vi "XW angle calib checker_Psi_k_PN.vi"(0 "XW_Calib_Map file path (dialog if empty)":path=path "C:/Documents and Settings/Paul Nathan/Desktop/XW Calib Map/XW angle calib checker/XW002_OH74.txt") -> (1 "Quantities that vary with Uref (epsilon, theta, k) (higher order method)":string="Uref (m/s)\teps1 (deg)\teps2 (deg)\tProbe zero err. (deg)\ttheta 1 (deg)\ttheta 2 (deg)\tk1\tk2\r\n0.5018157894736842\t6.6267533355295098\t-2.9096917617315157\t1.8585307868989971\t-71.8440498634698059\t62.9636877172930269\t0.6599332295131556\t0.5182677319056693\r\n0.9994315789473684\t-1.5238812538483015\t0.9867720938009503\t-0.2685545800236756\t-50.7967211983630804\t49.0160971121406277\t0.4477378321660210\t0.4147363151308795\r\n2.0002052631578948\t-0.7133248964583321\t0.8757082064818565\t0.0811916550117622\t-47.4142025982968249\t46.7238739777964795\t0.3482854524979783\t0.3208003585595113\r\n3.0007842105263158\t0.1760631838109192\t0.0773496663189750\t0.1267064250649471\t-46.5210606369966655\t46.4000168794064791\t0.3180701353043149\t0.2880980466431171\r\n3.9999473684210529\t0.1906487887884856\t-0.2531251578949707\t-0.0312381845532425\t-46.1290205114913973\t46.2520699692747428\t0.2973863116337985\t0.2724916341605894\r\n4.9998315789473686\t0.2282387696125578\t-0.2130683224321221\t0.0075852235902178\t-45.8252448288331848\t46.0312176850919527\t0.2848963782809627\t0.2591128097080996\r\n6.9997315789473680\t0.1263159354503486\t-0.1724714828642656\t-0.0230777737069585\t-45.2896437061695636\t45.4966612147379905\t0.2642800771604700\t0.2410224971037092\r\n9.0019315789473691\t-0.0565462004426682\t0.0773785766074348\t0.0104161880823833\t-44.8675096760090781\t45.0959281609883007\t0.2463064031896132\t0.2236365187658773\r\n10.9999736842105253\t-0.2539290822848189\t0.4859354251419680\t0.1160031714285746\t-44.4053231675819475\t44.4986166412718447\t0.2285399354877705\t0.2028480726593353\r\n13.0001684210526314\t-0.5118579225506322\t0.7409038885633648\t0.1145229830063663\t-44.0067920576490863\t43.9637273900855589\t0.2106532081178256\t0.1851715125746722\r\n15.0011421052631579\t-0.7550503383633475\t0.9105592735667922\t0.0777544676017224\t-43.6252625738814430\t43.5843363193315980\t0.1938872474806054\t0.1681952069880485\r\n")   [LabVIEW 2011]
uses:
  <vilib>/Utility/file.llb/Read From Spreadsheet File (DBL).vi
  <vilib>/Utility/file.llb/Read From Spreadsheet File (string).vi
  <vilib>/Analysis/polynomials.llb/Polynomial Plot (Range).vi
  <vilib>/Analysis/polynomials.llb/Polynomial Roots (DBL).vi
  <vilib>/Analysis/polynomials.llb/Polynomial Plot (Samples).vi
  <vilib>/Analysis/NI_AALBase.lvlib
  <vilib>/Analysis/NI_AALPro.lvlib
panel:
  out "No real roots for the set (i.e. poor dataset)":bool[](array[boolean])
  in  "Transfer query set control here":bool
  in  "Query set (alias)":i32
  out "Quartic tan(2e) function":cluster{dbl[], dbl[]}[](graph)
  out "Roots for e2 (2nd index angle set -1)":cdb[][](array[numeric])=[[-1.5312225140484632+0.0i, -5.7789881705260475+0.0i, 16.707412903025755+0.0i, 6.487596745899962+0.0i, 5.07875897772016+0.0i, 4.5149249062893295+0.0i, 3.8545352853829686+0.0i, 3.5396117006623347+0.0i, 3.2733530304807683+0.0i, 3.048630181958505+0.0i, 2.870340574754272+0.0i], [0.01605988720470126+0.9915361243519932i, 0.03085582521272682+0.993058906632486i, 0.0324524213798118+1.0004216780304256i, 0.032106706375471146+1.0043354071771722i, 0.031766443184513306+1.0060241435427537i, 0.03160334336742563+1.006724744418667i, 0.032056349283290625+1.0079772109676068i, 0.03221519106415766+1.0084528128807435i, 0.03283135973491863+1.008846021301184i, 0.033545476601848256+1.0094431819546548i, 0.033931484900126194+1.0099991970101188i], [0.01605988720470126-0.9915361243519932i, 0.03085582521272682-0.993058906632486i, 0.0324524213798118-1.0004216780304256i, 0.032106706375471146-1.0043354071771722i, 0.031766443184513306-1.0060241435427537i, 0.03160334336742563-1.006724744418667i, 0.032056349283290625-1.0079772109676068i, 0.03221519106415766-1.0084528128807435i, 0.03283135973491863-1.008846021301184i, 0.033545476601848256-1.0094431819546548i, 0.033931484900126194-1.0099991970101188i], [-0.10191810443911971+0.0i, 0.03445847280570573+0.0i, 0.030577507463478086+0.0i, 0.0027000192662819055+0.0i, -0.00883596479286893+0.0i, -0.007437624657217234+0.0i, -0.006020463221166247+0.0i, 0.0027010284330841834+0.0i, 0.016963973237675695+0.0i, 0.025868192292574817+0.0i, 0.03179522253597648+0.0i]]
  out "Roots for e1 (2nd index angle set- 1)":cdb[][](array[numeric])=[[-0.015920835836600956+0.9840410941913059i, 3.395480898493778+0.0i, -594.6858847661478+0.0i, -9.256262608165473+0.0i, -6.488582226964649+0.0i, -5.441866908194584+0.0i, -4.436840208641861+0.0i, -3.9198732443788966+0.0i, -3.5319472433943178+0.0i, -3.274664710498834+0.0i, -3.0804435614198376+0.0i], [-0.015920835836600956-0.9840410941913059i, -0.027443163981895065+0.9898767262763457i, -0.03214949692082573+0.9987358189508502i, -0.033633194220896445+1.0032718682899566i, -0.03351716383634002+1.004820829232972i, -0.033650835494892437+1.0058777923714683i, -0.033930025437022095+1.0072031374933277i, -0.034075572988984906+1.0080087857191546i, -0.034416949826886596+1.008784914915294i, -0.03463560472159067+1.009261191747309i, -0.03494277753284658+1.0096764982859878i], [0.6282192557965222+0.0i, -0.027443163981895065-0.9898767262763457i, -0.03214949692082573-0.9987358189508502i, -0.033633194220896445-1.0032718682899566i, -0.03351716383634002-1.004820829232972i, -0.033650835494892437-1.0058777923714683i, -0.033930025437022095-1.0072031374933277i, -0.034075572988984906-1.0080087857191546i, -0.034416949826886596-1.008784914915294i, -0.03463560472159067-1.009261191747309i, -0.03494277753284658-1.0096764982859878i], [0.23553334080037672+0.0i, -0.053243718596296244+0.0i, -0.024904883355210815+0.0i, 0.006145841875296093+0.0i, 0.00665499640364714+0.0i, 0.007967204590812788+0.0i, 0.004409286517190454+0.0i, -0.00197383731780742+0.0i, -0.008864029245855139+0.0i, -0.01786911363799798+0.0i, -0.02636233333348425+0.0i]]
  in  "Coefficient Constraint":cluster{"order":i32, "coefficient":dbl}[](array[cluster])
  in  "Ignore first n pts from calib.":i32
  out "Higher order effective angle method X plot data (each angle set separated by a column of zeros)":string="x_0\ty1_0\ty2_0\t\tx_1\ty1_1\ty2_1\t\tx_2\ty1_2\ty2_2\t\tx_3\ty1_3\ty2_3\t\tx_4\ty1_4\ty2_4\t\tx_5\ty1_5\ty2_5\t\tx_6\ty1_6\ty2_6\t\tx_7\ty1_7\ty2_7\t\tx_8\ty1_8\ty2_8\t\tx_9\ty1_9\ty2_9\t\tx_10\ty1_10\ty2_10\r\n-0.9999999999999999\t-0.9085791502544248\t-3.9630468181290452\t0.0000000000000000\t-0.9999999999999999\t0.1949143754370715\t-2.6536651485735696\t0.0000000000000000\t-0.9999999999999999\t0.5188418104065096\t-2.7107465604685741\t0.0000000000000000\t-0.9999999999999999\t0.6105115215521106\t-2.7972176259688553\t0.0000000000000000\t-0.9999999999999999\t0.6514204222508733\t-2.8375050105836368\t0.0000000000000000\t-0.9999999999999999\t0.6746558655695405\t-2.8404947938821206\t0.0000000000000000\t-0.9999999999999999\t0.7084619405900626\t-2.8035914112508933\t0.0000000000000000\t-0.9999999999999999\t0.7363342408659557\t-2.7810177224561561\t0.0000000000000000\t-0.9999999999999999\t0.7620888951136892\t-2.7288520875385447\t0.0000000000000000\t-0.9999999999999999\t0.7861588927941786\t-2.6856742001602751\t0.0000000000000000\t-0.9999999999999999\t0.8056811585366324\t-2.6550478856042679\t0.0000000000000000\r\n-0.8459634362504808\t-0.4625621144061756\t-2.8818271450789865\t0.0000000000000000\t-0.8459634362504808\t0.2815754544138509\t-2.1394999422469003\t0.0000000000000000\t-0.8459634362504808\t0.5527709767869218\t-2.2324745574527904\t0.0000000000000000\t-0.8459634362504808\t0.6382823976284421\t-2.2665818845631214\t0.0000000000000000\t-0.8459634362504808\t0.6788684735006610\t-2.2842367882197863\t0.0000000000000000\t-0.8459634362504808\t0.7029454921629841\t-2.2878897351586707\t0.0000000000000000\t-0.8459634362504808\t0.7360252511014151\t-2.2626966309367886\t0.0000000000000000\t-0.8459634362504808\t0.7617351722175852\t-2.2416920469763459\t0.0000000000000000\t-0.8432720672116305\t0.7844643868612465\t-2.1887614629441035\t0.0000000000000000\t-0.8432720672116305\t0.8038053956321515\t-2.1508294307461551\t0.0000000000000000\t-0.8432720672116305\t0.8196056618936665\t-2.1284563267855230\t0.0000000000000000\r\n-0.7028117712403573\t-0.0667229984385117\t-1.7990557676966663\t0.0000000000000000\t-0.7028117712403573\t0.3411211378733948\t-1.6837865113002857\t0.0000000000000000\t-0.7028117712403573\t0.5825100736406964\t-1.6930687846557417\t0.0000000000000000\t-0.7028117712403573\t0.6448979960495834\t-1.7825502259833412\t0.0000000000000000\t-0.7028117712403573\t0.6810359033183786\t-1.8105052193118192\t0.0000000000000000\t-0.7028117712403573\t0.7040869499204692\t-1.8110590099219335\t0.0000000000000000\t-0.7028117712403573\t0.7342043939074193\t-1.7929291162742504\t0.0000000000000000\t-0.7028117712403573\t0.7550109725157748\t-1.7756905349598751\t0.0000000000000000\t-0.7028117712403573\t0.7711095218508195\t-1.7384235052178580\t0.0000000000000000\t-0.7028117712403573\t0.7847492951756501\t-1.7045648544699419\t0.0000000000000000\t-0.7028117712403573\t0.7958199433613861\t-1.6859867806778905\t0.0000000000000000\r\n-0.5745611109571804\t-0.0376287976903837\t-1.5446740531776548\t0.0000000000000000\t-0.5745611109571804\t0.3599220910286302\t-1.3459064192482468\t0.0000000000000000\t-0.5745611109571804\t0.5655852803690335\t-1.3559695335879334\t0.0000000000000000\t-0.5745611109571804\t0.6247863747603235\t-1.3916622950809854\t0.0000000000000000\t-0.5745611109571804\t0.6553574621762963\t-1.4097043857813083\t0.0000000000000000\t-0.5745611109571804\t0.6735069299277736\t-1.4112094707533349\t0.0000000000000000\t-0.5745611109571804\t0.6949413208702192\t-1.4067266943759922\t0.0000000000000000\t-0.5745611109571804\t0.7105513693367174\t-1.3847598236387422\t0.0000000000000000\t-0.5745611109571804\t0.7218957685787146\t-1.3544132560361197\t0.0000000000000000\t-0.5766523484064272\t0.7309919560241551\t-1.3305928734680903\t0.0000000000000000\t-0.5745611109571804\t0.7384817158571489\t-1.3099108075871668\t0.0000000000000000\r\n-0.4610063144273182\t0.0412919475631363\t-1.0997890950007321\t0.0000000000000000\t-0.4610063144273182\t0.3770239497989202\t-0.9792680032688384\t0.0000000000000000\t-0.4610063144273182\t0.5367013693167687\t-1.0119826258435312\t0.0000000000000000\t-0.4610063144273182\t0.5743830527285835\t-1.0774202158722981\t0.0000000000000000\t-0.4610063144273182\t0.5979952814046342\t-1.0939710197186976\t0.0000000000000000\t-0.4667326950738877\t0.6116296380054032\t-1.0948501153158237\t0.0000000000000000\t-0.4610063144273182\t0.6279311798252735\t-1.0827733496154128\t0.0000000000000000\t-0.4610063144273182\t0.6377056286721594\t-1.0683619324969325\t0.0000000000000000\t-0.4610063144273182\t0.6452821120555695\t-1.0398621565011508\t0.0000000000000000\t-0.4629123289077153\t0.6520868780188794\t-1.0198362226727229\t0.0000000000000000\t-0.4629123289077153\t0.6571442461528323\t-1.0051143364341999\t0.0000000000000000\r\n-0.3689194771098271\t0.1044333744574640\t-0.7437632758411701\t0.0000000000000000\t-0.3689194771098271\t0.3703284183929321\t-0.7061988569542564\t0.0000000000000000\t-0.3689194771098271\t0.4814947359213608\t-0.7770192864712264\t0.0000000000000000\t-0.3689194771098271\t0.5088608177696153\t-0.8210529776089235\t0.0000000000000000\t-0.3635749763519443\t0.5263421036228286\t-0.8282138902172458\t0.0000000000000000\t-0.3689194771098271\t0.5331564790478260\t-0.8458290235908140\t0.0000000000000000\t-0.3689194771098271\t0.5437170073266897\t-0.8393399765706897\t0.0000000000000000\t-0.3689194771098271\t0.5501602814743358\t-0.8249109991926368\t0.0000000000000000\t-0.3689194771098271\t0.5563221043460842\t-0.7999971908211336\t0.0000000000000000\t-0.3689194771098271\t0.5623927525763176\t-0.7803547186651004\t0.0000000000000000\t-0.3689194771098271\t0.5671583051208874\t-0.7700855374663110\t0.0000000000000000\r\n-0.2718814121476857\t0.0255847727338301\t-0.6689751955611348\t0.0000000000000000\t-0.2718814121476857\t0.3106644522796246\t-0.5047454592362141\t0.0000000000000000\t-0.2718814121476857\t0.3962036651655259\t-0.5446172063124690\t0.0000000000000000\t-0.2718814121476857\t0.4082234758439587\t-0.5916721671054449\t0.0000000000000000\t-0.2718814121476857\t0.4191107855801626\t-0.5983889263646065\t0.0000000000000000\t-0.2718814121476857\t0.4242807676181213\t-0.6036578351430176\t0.0000000000000000\t-0.2718814121476857\t0.4289132363159743\t-0.6011772566633612\t0.0000000000000000\t-0.2718814121476857\t0.4344930216745795\t-0.5885638990500427\t0.0000000000000000\t-0.2718814121476857\t0.4407940406478280\t-0.5667386082032163\t0.0000000000000000\t-0.2718814121476857\t0.4466625036118104\t-0.5511317529698531\t0.0000000000000000\t-0.2718814121476857\t0.4513779468028263\t-0.5395864188016505\t0.0000000000000000\r\n-0.1761470268806888\t-0.0942490676366393\t-0.5868960272983509\t0.0000000000000000\t-0.1761470268806888\t0.2548185009347063\t-0.2645492620955306\t0.0000000000000000\t-0.1761470268806888\t0.3024751991218511\t-0.2921952683619167\t0.0000000000000000\t-0.1761470268806888\t0.2870434875402270\t-0.3500127136267793\t0.0000000000000000\t-0.1761470268806888\t0.2830095550319655\t-0.3828463334548899\t0.0000000000000000\t-0.1761470268806888\t0.2855455723517732\t-0.3809026465127626\t0.0000000000000000\t-0.1761470268806888\t0.2884644985637423\t-0.3799013981302747\t0.0000000000000000\t-0.1761470268806888\t0.2930495918311506\t-0.3699160983941475\t0.0000000000000000\t-0.1761470268806888\t0.2992247712103860\t-0.3541806551714389\t0.0000000000000000\t-0.1761470268806888\t0.3058374237252131\t-0.3408777024657876\t0.0000000000000000\t-0.1761470268806888\t0.3111246627753121\t-0.3320591164269514\t0.0000000000000000\r\n-0.0850270210113130\t-0.0504595050252811\t-0.2775995341357290\t0.0000000000000000\t-0.0850270210113130\t0.1736177181817981\t-0.0758426654882593\t0.0000000000000000\t-0.0850270210113130\t0.1727751104131255\t-0.1124460755508965\t0.0000000000000000\t-0.0850270210113130\t0.1397558723489909\t-0.1611761582181669\t0.0000000000000000\t-0.0850270210113130\t0.1364092384545839\t-0.1803971782800010\t0.0000000000000000\t-0.0850270210113130\t0.1330151029088564\t-0.1846382073328683\t0.0000000000000000\t-0.0850270210113130\t0.1336180079889946\t-0.1859543864792222\t0.0000000000000000\t-0.0850270210113130\t0.1391330147914122\t-0.1779026144672113\t0.0000000000000000\t-0.0881921819968595\t0.1468097530657032\t-0.1664128928822258\t0.0000000000000000\t-0.0850270210113130\t0.1533034947310865\t-0.1537657502004380\t0.0000000000000000\t-0.0850270210113130\t0.1602920927213465\t-0.1466312867329973\t0.0000000000000000\r\n0.0000000000000000\t-0.1396755488429087\t-0.1495552894031837\t0.0000000000000000\t0.0000000000000000\t0.1015398030851381\t0.0979907823209607\t0.0000000000000000\t0.0000000000000000\t0.0485713499475330\t0.0551796899852733\t0.0000000000000000\t0.0000000000000000\t0.0039204586603697\t0.0100793521533393\t0.0000000000000000\t0.0000000000000000\t-0.0123772694902811\t-0.0123048930616856\t0.0000000000000000\t0.0000000000000000\t-0.0158825708767742\t-0.0172400662126269\t0.0000000000000000\t0.0000000000000000\t-0.0185621834928470\t-0.0203971278636718\t0.0000000000000000\t0.0000000000000000\t-0.0117122957217886\t-0.0145134805930901\t0.0000000000000000\t-0.0015707976187244\t-0.0034205951378717\t-0.0026021495757281\t0.0000000000000000\t0.0000000000000000\t0.0051491403774043\t0.0063664317326143\t0.0000000000000000\t0.0000000000000000\t0.0119067452638700\t0.0115332438693104\t0.0000000000000000\r\n0.0834450784477064\t-0.0417648215636864\t0.1352429486294378\t0.0000000000000000\t0.0834450784477064\t-0.0776394529995262\t0.1668355133205353\t0.0000000000000000\t0.0834450784477064\t-0.1147770314630093\t0.1823015191280195\t0.0000000000000000\t0.0834450784477064\t-0.1518089738821856\t0.1616926063828080\t0.0000000000000000\t0.0834450784477064\t-0.1675177345562901\t0.1418323488914914\t0.0000000000000000\t0.0834450784477064\t-0.1743808906051748\t0.1396223268122237\t0.0000000000000000\t0.0834450784477064\t-0.1748799907332232\t0.1407817659046222\t0.0000000000000000\t0.0834450784477064\t-0.1711359562908112\t0.1443459528715696\t0.0000000000000000\t0.0834450784477064\t-0.1631451101745820\t0.1538692306045876\t0.0000000000000000\t0.0834450784477064\t-0.1562961885310737\t0.1594290597441742\t0.0000000000000000\t0.0834450784477064\t-0.1463689695846851\t0.1660732505077365\t0.0000000000000000\r\n0.1745279388943651\t-0.2504441955126037\t0.1552207836757285\t0.0000000000000000\t0.1745279388943651\t-0.1923048605897919\t0.3015431454828965\t0.0000000000000000\t0.1745279388943651\t-0.3118645832700102\t0.3060446247312193\t0.0000000000000000\t0.1745279388943651\t-0.3399045763763606\t0.3042221403451356\t0.0000000000000000\t0.1745279388943651\t-0.3591535093836093\t0.2969861016671120\t0.0000000000000000\t0.1745279388943651\t-0.3625352124879301\t0.2987758625039919\t0.0000000000000000\t0.1745279388943651\t-0.3625811847622155\t0.2987619180587648\t0.0000000000000000\t0.1761470268806888\t-0.3586700905175086\t0.3043173930134577\t0.0000000000000000\t0.1745279388943651\t-0.3487858594270737\t0.3125226906016907\t0.0000000000000000\t0.1745279388943651\t-0.3381938626612139\t0.3167839456066439\t0.0000000000000000\t0.1745279388943651\t-0.3288971373969858\t0.3213424951515983\t0.0000000000000000\r\n0.2701952220731489\t-0.4823610385730527\t0.1684170210190646\t0.0000000000000000\t0.2701952220731489\t-0.3941480974967655\t0.3747405534620119\t0.0000000000000000\t0.2685104627037557\t-0.5123196133813664\t0.4244954643928500\t0.0000000000000000\t0.2685104627037557\t-0.5622716481313378\t0.4320516895393265\t0.0000000000000000\t0.2685104627037557\t-0.5746725215951116\t0.4333475328171350\t0.0000000000000000\t0.2701952220731489\t-0.5761161656795665\t0.4382762721402697\t0.0000000000000000\t0.2701952220731489\t-0.5711564795303717\t0.4462115429854009\t0.0000000000000000\t0.2685104627037557\t-0.5637027508394487\t0.4500064910221563\t0.0000000000000000\t0.2685104627037557\t-0.5531821206069903\t0.4562858049551752\t0.0000000000000000\t0.2685104627037557\t-0.5410697161194152\t0.4598006047578997\t0.0000000000000000\t0.2685104627037557\t-0.5305871950835828\t0.4640535298803268\t0.0000000000000000\r\n0.3635749763519443\t-0.6862363241063577\t0.1938745671240703\t0.0000000000000000\t0.3671359250169842\t-0.6594497435504401\t0.4155995678888906\t0.0000000000000000\t0.3689194771098271\t-0.8062252804138840\t0.4942666230060676\t0.0000000000000000\t0.3671359250169842\t-0.8150435379645339\t0.5333980586374278\t0.0000000000000000\t0.3671359250169842\t-0.8025341705196405\t0.5488805679771741\t0.0000000000000000\t0.3689194771098271\t-0.8130451171136217\t0.5564687631683539\t0.0000000000000000\t0.3671359250169842\t-0.8041120781889549\t0.5656961795372176\t0.0000000000000000\t0.3671359250169842\t-0.7982752853845158\t0.5727446882583248\t0.0000000000000000\t0.3671359250169842\t-0.7840331881102651\t0.5783268868158106\t0.0000000000000000\t0.3671359250169842\t-0.7703712073294504\t0.5816443488942544\t0.0000000000000000\t0.3671359250169842\t-0.7586054072639649\t0.5859279656615510\t0.0000000000000000\r\n0.4629123289077153\t-0.8476294329786266\t0.2235614092068809\t0.0000000000000000\t0.4629123289077153\t-0.9492224197361369\t0.4327728553093401\t0.0000000000000000\t0.4610063144273182\t-0.9819378661710078\t0.5718021480660419\t0.0000000000000000\t0.4610063144273182\t-1.0553848834240576\t0.6055334918430288\t0.0000000000000000\t0.4610063144273182\t-1.0574404797332702\t0.6253666996480907\t0.0000000000000000\t0.4610063144273182\t-1.0556690478955482\t0.6393228823720644\t0.0000000000000000\t0.4610063144273182\t-1.0477195054982680\t0.6529818956214503\t0.0000000000000000\t0.4610063144273182\t-1.0344062288018556\t0.6626927832176096\t0.0000000000000000\t0.4610063144273182\t-1.0205105865152524\t0.6697752152893657\t0.0000000000000000\t0.4610063144273182\t-1.0056840847353361\t0.6738862961883090\t0.0000000000000000\t0.4667326950738877\t-0.9992094770597746\t0.6782936840236679\t0.0000000000000000\r\n0.5724736448682121\t-1.3899789264513560\t0.1020641173846400\t0.0000000000000000\t0.5724736448682121\t-1.2323317956367625\t0.4538004753460074\t0.0000000000000000\t0.5724736448682121\t-1.3238555928281337\t0.6021700169460663\t0.0000000000000000\t0.5724736448682121\t-1.3635980664653848\t0.6589555940191650\t0.0000000000000000\t0.5724736448682121\t-1.3598145734442184\t0.6847037690811968\t0.0000000000000000\t0.5724736448682121\t-1.3684754908238803\t0.7014719043851134\t0.0000000000000000\t0.5724736448682121\t-1.3561242322873066\t0.7226084437915833\t0.0000000000000000\t0.5724736448682121\t-1.3414409891263650\t0.7365615404721209\t0.0000000000000000\t0.5703899296732948\t-1.3202033688759527\t0.7473204528114626\t0.0000000000000000\t0.5703899296732948\t-1.3047561674071091\t0.7540053749349491\t0.0000000000000000\t0.5703899296732948\t-1.2856457129099557\t0.7602089334598410\t0.0000000000000000\r\n0.7004676747806673\t-2.2697364417842891\t-0.1308275547072091\t0.0000000000000000\t0.7004676747806673\t-1.6322660285466430\t0.4389604957859697\t0.0000000000000000\t0.7004676747806673\t-1.7125591635376343\t0.6186366367406101\t0.0000000000000000\t0.7004676747806673\t-1.7507849758841230\t0.6833036449657283\t0.0000000000000000\t0.7004676747806673\t-1.7532033361976842\t0.7149717797808454\t0.0000000000000000\t0.7004676747806673\t-1.7468810658722469\t0.7363863563633494\t0.0000000000000000\t0.6981287310371237\t-1.7323516588972048\t0.7628805858487009\t0.0000000000000000\t0.7004676747806673\t-1.7225575014273988\t0.7821105315579404\t0.0000000000000000\t0.6981287310371237\t-1.6962155420747351\t0.7969917434866054\t0.0000000000000000\t0.6981287310371237\t-1.6783350413415989\t0.8084591863151523\t0.0000000000000000\t0.6981287310371237\t-1.6580717599172035\t0.8184445444178572\t0.0000000000000000\r\n0.8432720672116305\t-2.2413583286537802\t-0.0361829804629510\t0.0000000000000000\t0.8432720672116305\t-2.3075415725227733\t0.3599602272717538\t0.0000000000000000\t0.8432720672116305\t-2.1691060617855422\t0.6115535237817370\t0.0000000000000000\t0.8432720672116305\t-2.2290412862152995\t0.6830463271258672\t0.0000000000000000\t0.8432720672116305\t-2.2222009266918268\t0.7182124425293464\t0.0000000000000000\t0.8379106495048978\t-2.2019648631264235\t0.7421134752332942\t0.0000000000000000\t0.8432720672116305\t-2.1971863462195551\t0.7681137807799585\t0.0000000000000000\t0.8432720672116305\t-2.1821977941933697\t0.7910287339996136\t0.0000000000000000\t0.8432720672116305\t-2.1597258190303488\t0.8104743841359477\t0.0000000000000000\t0.8432720672116305\t-2.1347740356153819\t0.8264250196496778\t0.0000000000000000\t0.8432720672116305\t-2.1122974634158354\t0.8411438740059636\t0.0000000000000000\r\n0.9999999999999999\t-2.8237734406173329\t-0.1791722171870904\t0.0000000000000000\t0.9999999999999999\t-2.6217506945340499\t0.3404580267525550\t0.0000000000000000\t0.9999999999999999\t-2.7652216719375038\t0.5776183997010226\t0.0000000000000000\t0.9999999999999999\t-2.7434622913910154\t0.6673214592086288\t0.0000000000000000\t0.9999999999999999\t-2.7691832771154199\t0.7016501297022305\t0.0000000000000000\t0.9999999999999999\t-2.7634005636598853\t0.7220453961815417\t0.0000000000000000\t0.9999999999999999\t-2.7441674751271026\t0.7453072103707526\t0.0000000000000000\t0.9999999999999999\t-2.7255665231484856\t0.7665049857410070\t0.0000000000000000\t0.9999999999999999\t-2.6957943045968502\t0.7883146132106904\t0.0000000000000000\t0.9999999999999999\t-2.6708083003892944\t0.8079886891481993\t0.0000000000000000\t0.9999999999999999\t-2.6439319990345118\t0.8268920789495620\t0.0000000000000000\r\n"
  out "E1, E2 maps for each method":string="E1' actual data (Volts)\tE2' actual data (Volts)\tE1' higher order eff. angle method (Volts)\tE2' higher order eff. angle method (Volts)\r\n2.3579666669999999\t2.9299833330000000\t2.3383503559788665\t2.9316284744959002\r\n2.3677166669999998\t2.9294583329999999\t2.3592701729486283\t2.9298814778055742\r\n2.4008333330000000\t2.9260500000000000\t2.4048236830520437\t2.9257250223026987\r\n2.4493749999999999\t2.9185666669999999\t2.4594505790418713\t2.9177220756629931\r\n2.5012333330000001\t2.9088250000000002\t2.5115913483381052\t2.9076529792842338\r\n2.5454750000000002\t2.8961416670000002\t2.5544939228716399\t2.8942399191403410\r\n2.5916916670000001\t2.8796666670000000\t2.5979496262689916\t2.8775059223987949\r\n2.6357833330000000\t2.8591916670000002\t2.6378890227350245\t2.8563540026666883\r\n2.6740083330000002\t2.8352249999999999\t2.6729624184416063\t2.8322389597734614\r\n2.7039083330000002\t2.8084750000000001\t2.7018303550309795\t2.8051956731962187\r\n2.7292333329999998\t2.7755916670000000\t2.7264793868299209\t2.7747012472666093\r\n2.7522583329999999\t2.7347416670000002\t2.7496761697964351\t2.7377544628056012\r\n2.7705500000000001\t2.6868083330000001\t2.7684960736541346\t2.6950384733553792\r\n2.7864583330000001\t2.6357333330000001\t2.7850102267006269\t2.6478961670718619\r\n2.7969249999999999\t2.5853166669999998\t2.7967509844150462\t2.5972697210789715\r\n2.8072916669999999\t2.5308250000000001\t2.8067764571536102\t2.5451810967499258\r\n2.8134833330000002\t2.4766949999999999\t2.8132596002773957\t2.4833141088915949\r\n2.8174833330000002\t2.4419083330000002\t2.8178884541640654\t2.4293442883413552\r\n2.8178166670000002\t2.4331749999999999\t2.8188839610583316\t2.4047536835037198\r\n2.3343583330000000\t2.8727916670000000\t2.3158879734420954\t2.8743595443189611\r\n2.3435000000000001\t2.8738916670000001\t2.3346533288434310\t2.8744167182193658\r\n2.3714750000000002\t2.8703249999999998\t2.3751365251972985\t2.8700709383334031\r\n2.4142416670000002\t2.8624833330000001\t2.4238198263324695\t2.8617459752350940\r\n2.4608750000000001\t2.8512000000000000\t2.4717792647178034\t2.8498721288557669\r\n2.5054500000000002\t2.8424999999999998\t2.5148485663699311\t2.8407023272977865\r\n2.5484416670000001\t2.8258666670000001\t2.5550039513135379\t2.8234453018600409\r\n2.5895250000000001\t2.8049416670000000\t2.5919002511243088\t2.8020074818932690\r\n2.6267416670000001\t2.7825500000000001\t2.6257747186158844\t2.7795390318909603\r\n2.6555416670000000\t2.7572416670000002\t2.6537006688968261\t2.7541545449172755\r\n2.6786083330000001\t2.7247833330000000\t2.6757295847117124\t2.7235750231381171\r\n2.7000750000000000\t2.6853333330000000\t2.6976016491294419\t2.6882208511098544\r\n2.7202500000000001\t2.6422333330000001\t2.7182867360527414\t2.6502011926536486\r\n2.7338249999999999\t2.5924333329999998\t2.7324792043794761\t2.6042743447956163\r\n2.7455750000000001\t2.5466750000000000\t2.7447152330790900\t2.5607784404159464\r\n2.7540749999999998\t2.4944783330000000\t2.7533725574405614\t2.5085053460411464\r\n2.7618916670000000\t2.4476916670000000\t2.7616548966630807\t2.4535044878158234\r\n2.7636250000000002\t2.4171916670000000\t2.7641303636212169\t2.4046965022006166\r\n2.7645749999999998\t2.4109500000000001\t2.7657590592939294\t2.3850742592889551\r\n2.3075791670000001\t2.8102583330000002\t2.2900992757661354\t2.8120202846450195\r\n2.3143783330000001\t2.8105000000000002\t2.3052373411332345\t2.8110647501828763\r\n2.3374916670000001\t2.8074750000000002\t2.3408120702512694\t2.8070707374121651\r\n2.3759583329999998\t2.8013416670000000\t2.3863658470930544\t2.8002834462357233\r\n2.4189250000000002\t2.7911000000000001\t2.4307625657786436\t2.7894306694399891\r\n2.4590999999999998\t2.7811166670000000\t2.4687541687154013\t2.7791719495193767\r\n2.4994583330000002\t2.7651666669999999\t2.5062212556052352\t2.7627114786855547\r\n2.5392833330000002\t2.7464333330000001\t2.5417904795306292\t2.7434336766945329\r\n2.5737250000000000\t2.7246416670000002\t2.5721200886672095\t2.7222775540908688\r\n2.6007166669999999\t2.6997666670000000\t2.5984393691881378\t2.6971844613138889\r\n2.6247250000000002\t2.6711583330000002\t2.6222284263428426\t2.6702787510211690\r\n2.6453000000000002\t2.6334916669999999\t2.6427817678884478\t2.6366281689017925\r\n2.6619666670000002\t2.5904416669999999\t2.6599037817614808\t2.5985140216684437\r\n2.6758500000000001\t2.5444249999999999\t2.6743812861950405\t2.5563365634294906\r\n2.6868249999999998\t2.5016850000000002\t2.6858800185168428\t2.5157277834205090\r\n2.6947916670000001\t2.4541700000000000\t2.6941400582634114\t2.4675550084744655\r\n2.7006916670000001\t2.4125916670000000\t2.7005295928331581\t2.4168745382417525\r\n2.7041916669999999\t2.3881000000000001\t2.7045660651345798\t2.3754795919178897\r\n2.7053166670000000\t2.3835083330000000\t2.7066081675391604\t2.3603966859582410\r\n2.2740350000000000\t2.7394500000000002\t2.2592353460317391\t2.7411826499505429\r\n2.2802375000000001\t2.7401583330000001\t2.2708863077094392\t2.7407401618922655\r\n2.2992593330000002\t2.7379166669999999\t2.3018633452963102\t2.7375151626217229\r\n2.3320333330000000\t2.7315749999999999\t2.3417254197323403\t2.7306160526915919\r\n2.3698583329999998\t2.7217166669999999\t2.3814274565447313\t2.7199466119961460\r\n2.4067666669999999\t2.7124750000000000\t2.4162716901086929\t2.7104369685913996\r\n2.4441916670000001\t2.6973583329999999\t2.4506487990414483\t2.6948099367453247\r\n2.4818250000000002\t2.6800666670000002\t2.4841929985006939\t2.6773927754172049\r\n2.5130499999999998\t2.6580416670000000\t2.5121447029676571\t2.6554016487178655\r\n2.5383499999999999\t2.6351333330000002\t2.5363137470211590\t2.6324570264792277\r\n2.5605583329999999\t2.6081249999999998\t2.5580235188590832\t2.6077087089170816\r\n2.5799750000000001\t2.5730083330000002\t2.5777160943799244\t2.5759559394444471\r\n2.5960666670000001\t2.5331666670000001\t2.5939200220338292\t2.5416134066039042\r\n2.6095083330000000\t2.4905450000000000\t2.6077560275977389\t2.5028929061626579\r\n2.6199750000000002\t2.4518916669999999\t2.6189430250224723\t2.4659864166354399\r\n2.6276833329999998\t2.4097916669999999\t2.6270535829437507\t2.4216415685885599\r\n2.6343500000000000\t2.3747750000000001\t2.6341924724784342\t2.3773936133675067\r\n2.6365666669999999\t2.3542083329999999\t2.6370115771767688\t2.3418766992389477\r\n2.6372249999999999\t2.3495416670000000\t2.6384940165840556\t2.3296455946375980\r\n2.2321166670000001\t2.6560999999999999\t2.2202101663833709\t2.6578836922781353\r\n2.2376083329999998\t2.6560333329999999\t2.2286043562002589\t2.6566140989136295\r\n2.2525750000000002\t2.6530250000000000\t2.2537015862099481\t2.6526936866308528\r\n2.2800241670000001\t2.6478999999999999\t2.2880886028809035\t2.6465401675612070\r\n2.3128224999999998\t2.6395000000000000\t2.3237292296665646\t2.6377331025544257\r\n2.3450083330000000\t2.6305749999999999\t2.3544433903813884\t2.6284150669358177\r\n2.3794666670000000\t2.6172666670000000\t2.3858891342469701\t2.6146533928379920\r\n2.4135749999999998\t2.6010249999999999\t2.4161571994053390\t2.5984478179293506\r\n2.4428333329999998\t2.5811833329999998\t2.4420854184734901\t2.5787888873502567\r\n2.4661166670000001\t2.5598083329999999\t2.4640734865814595\t2.5576545635213841\r\n2.4855499999999999\t2.5341833330000001\t2.4834304287479552\t2.5345096975866337\r\n2.5037333330000000\t2.5027591669999998\t2.5014677538275563\t2.5063743788185424\r\n2.5192749999999999\t2.4664025000000001\t2.5175482691966780\t2.4747007316821454\r\n2.5313500000000002\t2.4283833330000002\t2.5298423214509862\t2.4401875997107205\r\n2.5405500000000001\t2.3935749999999998\t2.5392317193639520\t2.4064660035973326\r\n2.5480333329999998\t2.3577916669999999\t2.5471697666667450\t2.3676313057223175\r\n2.5532666669999999\t2.3286416669999999\t2.5528945334315658\t2.3294278068141319\r\n2.5558833330000001\t2.3118500000000002\t2.5564004938563545\t2.2994994849500370\r\n2.5566333330000002\t2.3058500000000000\t2.5579639991190097\t2.2900290779522594\r\n2.1775000000000002\t2.5542500000000001\t2.1701290194757532\t2.5556156338827889\r\n2.1830250000000002\t2.5535416670000002\t2.1752481019937617\t2.5539334836982759\r\n2.1960166669999999\t2.5513249999999998\t2.1948604897554085\t2.5508994495111712\r\n2.2165416670000000\t2.5454166670000000\t2.2222903772082740\t2.5445722334409013\r\n2.2438583329999999\t2.5389666670000000\t2.2514025040047851\t2.5381504130275676\r\n2.2702916670000000\t2.5302500000000001\t2.2785020167160894\t2.5282010087853983\r\n2.2996759999999998\t2.5183249999999999\t2.3059413806125288\t2.5160476008130059\r\n2.3292166669999999\t2.5031358330000000\t2.3319406385634860\t2.5009302356624836\r\n2.3559749999999999\t2.4863166670000001\t2.3557911966161349\t2.4844811643729878\r\n2.3760916669999999\t2.4666950000000001\t2.3749772752480527\t2.4653454480928079\r\n2.3937666670000000\t2.4444666669999999\t2.3922038783313639\t2.4448336972957656\r\n2.4100833330000002\t2.4163500000000000\t2.4082944010114500\t2.4200098586485472\r\n2.4243666670000001\t2.3856666670000002\t2.4226408161080473\t2.3922233075293238\r\n2.4357583329999999\t2.3528916670000002\t2.4343636777940874\t2.3621283582934387\r\n2.4436166670000001\t2.3235916670000001\t2.4422582076255481\t2.3334807173521246\r\n2.4501916669999999\t2.2949333329999999\t2.4491471702855887\t2.3006666252684655\r\n2.4553416669999999\t2.2722166669999999\t2.4552254746024911\t2.2697560352357065\r\n2.4578833329999998\t2.2576166670000002\t2.4580452103119077\t2.2478443043679976\r\n2.4582000000000002\t2.2499500000000001\t2.4595552996241476\t2.2415854888313329\r\n2.1434833329999998\t2.4913675000000000\t2.1388703075628865\t2.4927400161895208\r\n2.1502083330000001\t2.4918591669999999\t2.1431099469176700\t2.4923198608678301\r\n2.1616333330000002\t2.4891800000000002\t2.1588467025521054\t2.4887143147054815\r\n2.1792166669999999\t2.4840724999999999\t2.1827500400170079\t2.4832433478433602\r\n2.2021833329999998\t2.4772233330000000\t2.2088200252962240\t2.4753652240812771\r\n2.2257333330000000\t2.4692133329999999\t2.2340989619211231\t2.4674320198639599\r\n2.2519166670000001\t2.4583266670000001\t2.2573987264012101\t2.4565234278259576\r\n2.2789400000000000\t2.4450916669999998\t2.2813113555610403\t2.4428068912367107\r\n2.3021067500000001\t2.4280249999999999\t2.3023811038298891\t2.4267895055529904\r\n2.3218883330000000\t2.4108833330000001\t2.3211207830190337\t2.4103615983426550\r\n2.3376666670000001\t2.3902916670000001\t2.3367052351734290\t2.3912490791293921\r\n2.3533249999999999\t2.3650166669999999\t2.3517208567333325\t2.3687063915906279\r\n2.3658250000000001\t2.3365333330000002\t2.3637825665278984\t2.3430220401927895\r\n2.3771583330000001\t2.3082500000000001\t2.3760663951051386\t2.3170506850911354\r\n2.3848583329999999\t2.2828416670000000\t2.3833188930501366\t2.2906883720483218\r\n2.3908583330000002\t2.2581416669999999\t2.3902597246905519\t2.2620510652975150\r\n2.3955750000000000\t2.2385083330000000\t2.3951605612875402\t2.2347724676556395\r\n2.3980583329999998\t2.2255333330000000\t2.3982430721836430\t2.2161551624453124\r\n2.3979333330000001\t2.2170083329999999\t2.3991986886511989\t2.2115758068653273\r\n2.1050916669999999\t2.4168500000000002\t2.1031063962079748\t2.4184506588112717\r\n2.1117916669999999\t2.4177083330000002\t2.1055858580074953\t2.4177188174051123\r\n2.1217166669999998\t2.4152583330000001\t2.1179118773200525\t2.4148584235364052\r\n2.1360083329999999\t2.4109500000000001\t2.1372275909775755\t2.4098137791561305\r\n2.1542916669999999\t2.4042833330000000\t2.1586888726529172\t2.4021899140704828\r\n2.1732416670000001\t2.3967083329999999\t2.1788271310352627\t2.3950610646593389\r\n2.1953499999999999\t2.3868499999999999\t2.1998726202469192\t2.3843109990040028\r\n2.2187583329999998\t2.3741666669999999\t2.2221484743301518\t2.3734655585315605\r\n2.2397000000000000\t2.3594166670000001\t2.2405824645436310\t2.3588524311755443\r\n2.2565833330000000\t2.3436249999999998\t2.2575547029220413\t2.3444593128731412\r\n2.2699833329999999\t2.3238916669999998\t2.2703340867252422\t2.3263376321193308\r\n2.2846758330000001\t2.3031166669999998\t2.2844236525152906\t2.3070234980919864\r\n2.2971474999999999\t2.2791250000000001\t2.2957341711881858\t2.2849086800034519\r\n2.3069916670000001\t2.2548499999999998\t2.3047340741860558\t2.2607567907770889\r\n2.3146800000000001\t2.2347333329999999\t2.3129294552874535\t2.2395960527336158\r\n2.3208058330000001\t2.2148750000000001\t2.3196459325088279\t2.2160846035695516\r\n2.3247091670000000\t2.1991000000000001\t2.3240772720804843\t2.1942160777261441\r\n2.3268333330000002\t2.1878750000000000\t2.3264876888333275\t2.1800156722641155\r\n2.3271250000000001\t2.1803583330000000\t2.3289343815238182\t2.1785288618302885\r\n2.0602083329999998\t2.3236666669999999\t2.0626720498635471\t2.3254667149933739\r\n2.0647416669999998\t2.3234916669999999\t2.0603578405384124\t2.3223407345237268\r\n2.0721750000000001\t2.3222749999999999\t2.0687369797223232\t2.3228151932054719\r\n2.0817916670000001\t2.3177083330000001\t2.0790309931676458\t2.3155822498434677\r\n2.0951333330000002\t2.3128166669999999\t2.0960300617523631\t2.3114415975864317\r\n2.1082666670000001\t2.3056999999999999\t2.1102045261773608\t2.3038554567246394\r\n2.1244999999999998\t2.2963916670000000\t2.1264836177437187\t2.2942966064052577\r\n2.1421666670000001\t2.2852583329999998\t2.1456055329825201\t2.2861110610925035\r\n2.1578333330000001\t2.2717583330000002\t2.1600330708935993\t2.2727610822130821\r\n2.1720666670000002\t2.2582416670000001\t2.1747041296043985\t2.2610336823042854\r\n2.1853250000000002\t2.2438083330000000\t2.1861316598790252\t2.2464437935778672\r\n2.1978916669999999\t2.2268249999999998\t2.1971209732448242\t2.2295584474779031\r\n2.2085750000000002\t2.2084250000000001\t2.2080460882958683\t2.2127115999283027\r\n2.2177166669999999\t2.1911749999999999\t2.2142151042228972\t2.1919024572594381\r\n2.2262333330000001\t2.1776583330000001\t2.2263180586584856\t2.1801952510387896\r\n2.2299083330000000\t2.1629583330000002\t2.2288885158442500\t2.1607837959550262\r\n2.2349833330000002\t2.1523083330000001\t2.2345163014586076\t2.1474263279081578\r\n2.2355416670000001\t2.1430333330000000\t2.2362468566696942\t2.1389030046037796\r\n2.2367249999999999\t2.1377166669999998\t2.2372400818313447\t2.1389112820815122\r\n2.0031583330000000\t2.1960250000000001\t2.0081588878691332\t2.1976404350378567\r\n2.0045999999999999\t2.1949000000000001\t2.0039875824271043\t2.1949519062093539\r\n2.0074833330000001\t2.1930499999999999\t2.0035360947586591\t2.1920273716756120\r\n2.0119250000000002\t2.1903666670000002\t2.0059225051618341\t2.1871525078010192\r\n2.0170333330000001\t2.1855416669999999\t2.0130992447705691\t2.1837401331474653\r\n2.0236333329999998\t2.1812083329999998\t2.0220456271373544\t2.1809144764269583\r\n2.0313416670000000\t2.1737250000000001\t2.0294429076397300\t2.1722597936161585\r\n2.0397916669999998\t2.1643750000000002\t2.0401618078465042\t2.1651474904973740\r\n2.0486416670000001\t2.1545083329999999\t2.0504270297604310\t2.1568028159743058\r\n2.0583250000000000\t2.1458750000000002\t2.0630700092522662\t2.1512481057232393\r\n2.0650333330000001\t2.1343250000000000\t2.0658101545565470\t2.1361673035829787\r\n2.0748666670000002\t2.1247666669999998\t2.0784776331032386\t2.1292989369291262\r\n2.0832999999999999\t2.1147499999999999\t2.0860819442264806\t2.1178731597677332\r\n2.0910083330000000\t2.1058833330000000\t2.0914336463851146\t2.1061634918419938\r\n2.0972083330000002\t2.0990750000000000\t2.0957559686116736\t2.0962651165977686\r\n2.1020249999999998\t2.0923416669999999\t2.1017074652566765\t2.0891387266941703\r\n2.1062166670000000\t2.0873249999999999\t2.1060469717271464\t2.0837032208741397\r\n2.1089833329999998\t2.0837249999999998\t2.1045492973006641\t2.0786918971248558\r\n2.1112916670000001\t2.0818833329999999\t2.1139565471797277\t2.0860855205854398\r\n1.9603916669999999\t2.1036166669999998\t1.9575788692332172\t2.0993450708002266\r\n1.9639500000000001\t2.1090666670000000\t1.9638754448679856\t2.1081859723393812\r\n1.9648583330000000\t2.1094166670000001\t1.9718851848727175\t2.1172539074645957\r\n1.9647833330000000\t2.1051083330000000\t1.9657952573738435\t2.1074171893413549\r\n1.9650666670000001\t2.0985000000000000\t1.9656095922632972\t2.1021547889051000\r\n1.9663583330000001\t2.0928749999999998\t1.9684471598944637\t2.0990573928252814\r\n1.9673416669999999\t2.0863999999999998\t1.9645307106499681\t2.0859254402479026\r\n1.9705333330000001\t2.0802000000000000\t1.9630488586900885\t2.0738583707786344\r\n1.9759333330000000\t2.0757916669999998\t1.9737393912563916\t2.0734453420996939\r\n1.9812083330000001\t2.0706166669999999\t1.9787210752237252\t2.0669094436170874\r\n1.9869916670000001\t2.0655083329999999\t1.9950392155024053\t2.0708341977011009\r\n1.9886999999999999\t2.0561500000000001\t1.9926978447339572\t2.0566333134353028\r\n1.9939833330000001\t2.0512166669999998\t1.9955596231884831\t2.0480645848067485\r\n1.9985250000000001\t2.0469833330000000\t2.0001865052800407\t2.0431501331204016\r\n2.0033666669999999\t2.0445500000000001\t2.0080080426725826\t2.0425933159008554\r\n2.0072916670000001\t2.0421833330000001\t2.0054975528492105\t2.0360097778954516\r\n2.0103749999999998\t2.0405666669999998\t2.0000078973718614\t2.0297592737895616\r\n2.0160833330000001\t2.0411750000000000\t2.0175964547338414\t2.0441717971286488\r\n2.0187750000000002\t2.0414916669999998\t2.0219756231439270\t2.0504677149198711\r\n"
  out "Effective angle X plot_":cluster{dbl[], dbl[]}[](graph)=[{[-0.9999999999999999, -0.8459634362504808, -0.7028117712403573, -0.5745611109571804, -0.46100631442731815, -0.3689194771098271, -0.2718814121476857, -0.17614702688068878, -0.08502702101131297, 0.0, 0.0834450784477064, 0.17452793889436508, 0.26851046270375567, 0.3689194771098271, 0.46100631442731815, 0.5724736448682121, 0.7004676747806673, 0.8432720672116305, 0.9999999999999999], [0.5188418104065096, 0.5527709767869218, 0.5825100736406964, 0.5655852803690335, 0.5367013693167687, 0.4814947359213608, 0.3962036651655259, 0.30247519912185106, 0.17277511041312554, 0.04857134994753296, -0.11477703146300927, -0.31186458327001015, -0.5123196133813664, -0.806225280413884, -0.9819378661710078, -1.3238555928281337, -1.7125591635376343, -2.169106061785542, -2.765221671937504]}, {[-0.9999999999999999, -0.8459634362504808, -0.7028117712403573, -0.5745611109571804, -0.46100631442731815, -0.3689194771098271, -0.2718814121476857, -0.17614702688068878, -0.08502702101131297, 0.0, 0.0834450784477064, 0.17452793889436508, 0.26851046270375567, 0.3689194771098271, 0.46100631442731815, 0.5724736448682121, 0.7004676747806673, 0.8432720672116305, 0.9999999999999999], [-2.710746560468574, -2.2324745574527904, -1.6930687846557417, -1.3559695335879334, -1.0119826258435312, -0.7770192864712264, -0.544617206312469, -0.29219526836191667, -0.1124460755508965, 0.05517968998527327, 0.1823015191280195, 0.30604462473121935, 0.42449546439284996, 0.49426662300606755, 0.5718021480660419, 0.6021700169460663, 0.6186366367406101, 0.611553523781737, 0.5776183997010226]}, {[-0.9999999999999999, -0.8459634362504808, -0.7028117712403573, -0.5745611109571804, -0.46100631442731815, -0.3689194771098271, -0.2718814121476857, -0.17614702688068878, -0.08502702101131297, 0.0, 0.0834450784477064, 0.17452793889436508, 0.26851046270375567, 0.3689194771098271, 0.46100631442731815, 0.5724736448682121, 0.7004676747806673, 0.8432720672116305, 0.9999999999999999], [0.5019896305748247, 0.5792706211983509, 0.6016610033211529, 0.5812787539845564, 0.5313291123028853, 0.4688203592849761, 0.3816276240927678, 0.2741639698201763, 0.15209777501455385, 0.020792179522619556, -0.12440427224684161, -0.30136038420878597, -0.5041583453049925, -0.7435017841584199, -0.9836035435327022, -1.300599354618582, -1.7002055402395368, -2.1909817665541462, -2.7841533319516247]}, {[-0.9999999999999999, -0.8459634362504808, -0.7028117712403573, -0.5745611109571804, -0.46100631442731815, -0.3689194771098271, -0.2718814121476857, -0.17614702688068878, -0.08502702101131297, 0.0, 0.0834450784477064, 0.17452793889436508, 0.26851046270375567, 0.3689194771098271, 0.46100631442731815, 0.5724736448682121, 0.7004676747806673, 0.8432720672116305, 0.9999999999999999], [-2.7754536431394143, -2.1968375982636825, -1.707127164891374, -1.3076789676725484, -0.9849942600134655, -0.7446882768884536, -0.5121759440962987, -0.30361736510901655, -0.12432862939743507, 0.026066724526630464, 0.1577965612831473, 0.28364140853636527, 0.3938612873900718, 0.4895873414882753, 0.5573717280147601, 0.6138122549836776, 0.644026852354821, 0.6340896215868704, 0.5701968170808946]}]
  out "Variation of tangential cooling coefficient k with speed":cluster{dbl[], dbl[]}[](graph)=[{[0.5018157894736842, 0.9994315789473684, 2.000205263157895, 3.000784210526316, 3.999947368421053, 4.999831578947369, 6.999731578947368, 9.001931578947369, 10.999973684210525, 13.000168421052631, 15.001142105263158], [0.6599332295131556, 0.447737832166021, 0.34828545249797827, 0.3180701353043149, 0.2973863116337985, 0.2848963782809627, 0.26428007716047, 0.24630640318961325, 0.22853993548777052, 0.21065320811782565, 0.19388724748060543]}, {[0.5018157894736842, 0.9994315789473684, 2.000205263157895, 3.000784210526316, 3.999947368421053, 4.999831578947369, 6.999731578947368, 9.001931578947369, 10.999973684210525, 13.000168421052631, 15.001142105263158], [0.5182677319056693, 0.4147363151308795, 0.32080035855951133, 0.28809804664311706, 0.2724916341605894, 0.2591128097080996, 0.24102249710370924, 0.2236365187658773, 0.20284807265933533, 0.18517151257467218, 0.1681952069880485]}]
  out "Probe zero alignment error_":cluster{dbl[], dbl[]}(graph)={[0.5018157894736842, 0.9994315789473684, 2.000205263157895, 3.000784210526316, 3.999947368421053, 4.999831578947369, 6.999731578947368, 9.001931578947369, 10.999973684210525, 13.000168421052631, 15.001142105263158], [1.858530786898997, -0.2685545800236756, 0.08119165501176223, 0.1267064250649471, -0.031238184553242537, 0.007585223590217849, -0.0230777737069585, 0.010416188082383288, 0.11600317142857455, 0.11452298300636626, 0.07775446760172239]}
  out "Effective angle variation with speed_":cluster{dbl[], dbl[]}[](graph)=[{[0.5018157894736842, 0.9994315789473684, 2.000205263157895, 3.000784210526316, 3.999947368421053, 4.999831578947369, 6.999731578947368, 9.001931578947369, 10.999973684210525, 13.000168421052631, 15.001142105263158], [-71.8440498634698, -50.79672119836308, -47.414202598296825, -46.521060636996665, -46.1290205114914, -45.825244828833185, -45.289643706169564, -44.86750967600908, -44.40532316758195, -44.006792057649086, -43.62526257388144]}, {[0.5018157894736842, 0.9994315789473684, 2.000205263157895, 3.000784210526316, 3.999947368421053, 4.999831578947369, 6.999731578947368, 9.001931578947369, 10.999973684210525, 13.000168421052631, 15.001142105263158], [62.96368771729303, 49.01609711214063, 46.72387397779648, 46.40001687940648, 46.25206996927474, 46.03121768509195, 45.49666121473799, 45.0959281609883, 44.498616641271845, 43.96372739008556, 43.5843363193316]}]
  out "Wire angle error with speed_":cluster{dbl[], dbl[]}[](graph)=[{[0.5018157894736842, 0.9994315789473684, 2.000205263157895, 3.000784210526316, 3.999947368421053, 4.999831578947369, 6.999731578947368, 9.001931578947369, 10.999973684210525, 13.000168421052631, 15.001142105263158], [6.62675333552951, -1.5238812538483015, -0.7133248964583321, 0.17606318381091918, 0.19064878878848562, 0.22823876961255776, 0.12631593545034855, -0.05654620044266824, -0.25392908228481886, -0.5118579225506322, -0.7550503383633475]}, {[0.5018157894736842, 0.9994315789473684, 2.000205263157895, 3.000784210526316, 3.999947368421053, 4.999831578947369, 6.999731578947368, 9.001931578947369, 10.999973684210525, 13.000168421052631, 15.001142105263158], [-2.9096917617315157, 0.9867720938009503, 0.8757082064818565, 0.077349666318975, -0.2531251578949707, -0.21306832243212206, -0.17247148286426556, 0.07737857660743482, 0.48593542514196797, 0.7409038885633648, 0.9105592735667922]}]
  out "E1', E2' map synthesized from effective angle methods LS fits":cluster{dbl[], dbl[]}[](graph)=[{[2.357966667, 2.367716667, 2.400833333, 2.449375, 2.501233333, 2.545475, 2.591691667, 2.635783333, 2.674008333, 2.703908333, 2.729233333, 2.752258333, 2.77055, 2.786458333, 2.796925, 2.807291667, 2.813483333, 2.817483333, 2.817816667, 2.334358333, 2.3435, 2.371475, 2.414241667, 2.460875, 2.50545, 2.548441667, 2.589525, 2.626741667, 2.655541667, 2.678608333, 2.700075, 2.72025, 2.733825, 2.745575, 2.754075, 2.761891667, 2.763625, 2.764575, 2.307579167, 2.314378333, 2.337491667, 2.375958333, 2.418925, 2.4591, 2.499458333, 2.539283333, 2.573725, 2.600716667, 2.624725, 2.6453, 2.661966667, 2.67585, 2.686825, 2.694791667, 2.700691667, 2.704191667, 2.705316667, 2.274035, 2.2802375, 2.299259333, 2.332033333, 2.369858333, 2.406766667, 2.444191667, 2.481825, 2.51305, 2.53835, 2.560558333, 2.579975, 2.596066667, 2.609508333, 2.619975, 2.627683333, 2.63435, 2.636566667, 2.637225, 2.232116667, 2.237608333, 2.252575, 2.280024167, 2.3128225, 2.345008333, 2.379466667, 2.413575, 2.442833333, 2.466116667, 2.48555, 2.503733333, 2.519275, 2.53135, 2.54055, 2.548033333, 2.553266667, 2.555883333, 2.556633333, 2.1775, 2.183025, 2.196016667, 2.216541667, 2.243858333, 2.270291667, 2.299676, 2.329216667, 2.355975, 2.376091667, 2.393766667, 2.410083333, 2.424366667, 2.435758333, 2.443616667, 2.450191667, 2.455341667, 2.457883333, 2.4582, 2.143483333, 2.150208333, 2.161633333, 2.179216667, 2.202183333, 2.225733333, 2.251916667, 2.27894, 2.30210675, 2.321888333, 2.337666667, 2.353325, 2.365825, 2.377158333, 2.384858333, 2.390858333, 2.395575, 2.398058333, 2.397933333, 2.105091667, 2.111791667, 2.121716667, 2.136008333, 2.154291667, 2.173241667, 2.19535, 2.218758333, 2.2397, 2.256583333, 2.269983333, 2.284675833, 2.2971475, 2.306991667, 2.31468, 2.320805833, 2.324709167, 2.326833333, 2.327125, 2.060208333, 2.064741667, 2.072175, 2.081791667, 2.095133333, 2.108266667, 2.1245, 2.142166667, 2.157833333, 2.172066667, 2.185325, 2.197891667, 2.208575, 2.217716667, 2.226233333, 2.229908333, 2.234983333, 2.235541667, 2.236725, 2.003158333, 2.0046, 2.007483333, 2.011925, 2.017033333, 2.023633333, 2.031341667, 2.039791667, 2.048641667, 2.058325, 2.065033333, 2.074866667, 2.0833, 2.091008333, 2.097208333, 2.102025, 2.106216667, 2.108983333, 2.111291667, 1.960391667, 1.96395, 1.964858333, 1.964783333, 1.965066667, 1.966358333, 1.967341667, 1.970533333, 1.975933333, 1.981208333, 1.986991667, 1.9887, 1.993983333, 1.998525, 2.003366667, 2.007291667, 2.010375, 2.016083333, 2.018775], [2.929983333, 2.929458333, 2.92605, 2.918566667, 2.908825, 2.896141667, 2.879666667, 2.859191667, 2.835225, 2.808475, 2.775591667, 2.734741667, 2.686808333, 2.635733333, 2.585316667, 2.530825, 2.476695, 2.441908333, 2.433175, 2.872791667, 2.873891667, 2.870325, 2.862483333, 2.8512, 2.8425, 2.825866667, 2.804941667, 2.78255, 2.757241667, 2.724783333, 2.685333333, 2.642233333, 2.592433333, 2.546675, 2.494478333, 2.447691667, 2.417191667, 2.41095, 2.810258333, 2.8105, 2.807475, 2.801341667, 2.7911, 2.781116667, 2.765166667, 2.746433333, 2.724641667, 2.699766667, 2.671158333, 2.633491667, 2.590441667, 2.544425, 2.501685, 2.45417, 2.412591667, 2.3881, 2.383508333, 2.73945, 2.740158333, 2.737916667, 2.731575, 2.721716667, 2.712475, 2.697358333, 2.680066667, 2.658041667, 2.635133333, 2.608125, 2.573008333, 2.533166667, 2.490545, 2.451891667, 2.409791667, 2.374775, 2.354208333, 2.349541667, 2.6561, 2.656033333, 2.653025, 2.6479, 2.6395, 2.630575, 2.617266667, 2.601025, 2.581183333, 2.559808333, 2.534183333, 2.502759167, 2.4664025, 2.428383333, 2.393575, 2.357791667, 2.328641667, 2.31185, 2.30585, 2.55425, 2.553541667, 2.551325, 2.545416667, 2.538966667, 2.53025, 2.518325, 2.503135833, 2.486316667, 2.466695, 2.444466667, 2.41635, 2.385666667, 2.352891667, 2.323591667, 2.294933333, 2.272216667, 2.257616667, 2.24995, 2.4913675, 2.491859167, 2.48918, 2.4840725, 2.477223333, 2.469213333, 2.458326667, 2.445091667, 2.428025, 2.410883333, 2.390291667, 2.365016667, 2.336533333, 2.30825, 2.282841667, 2.258141667, 2.238508333, 2.225533333, 2.217008333, 2.41685, 2.417708333, 2.415258333, 2.41095, 2.404283333, 2.396708333, 2.38685, 2.374166667, 2.359416667, 2.343625, 2.323891667, 2.303116667, 2.279125, 2.25485, 2.234733333, 2.214875, 2.1991, 2.187875, 2.180358333, 2.323666667, 2.323491667, 2.322275, 2.317708333, 2.312816667, 2.3057, 2.296391667, 2.285258333, 2.271758333, 2.258241667, 2.243808333, 2.226825, 2.208425, 2.191175, 2.177658333, 2.162958333, 2.152308333, 2.143033333, 2.137716667, 2.196025, 2.1949, 2.19305, 2.190366667, 2.185541667, 2.181208333, 2.173725, 2.164375, 2.154508333, 2.145875, 2.134325, 2.124766667, 2.11475, 2.105883333, 2.099075, 2.092341667, 2.087325, 2.083725, 2.081883333, 2.103616667, 2.109066667, 2.109416667, 2.105108333, 2.0985, 2.092875, 2.0864, 2.0802, 2.075791667, 2.070616667, 2.065508333, 2.05615, 2.051216667, 2.046983333, 2.04455, 2.042183333, 2.040566667, 2.041175, 2.041491667]}, {[2.3383503559788665, 2.3592701729486283, 2.4048236830520437, 2.4594505790418713, 2.511591348338105, 2.55449392287164, 2.5979496262689916, 2.6378890227350245, 2.6729624184416063, 2.7018303550309795, 2.726479386829921, 2.749676169796435, 2.7684960736541346, 2.785010226700627, 2.796750984415046, 2.8067764571536102, 2.8132596002773957, 2.8178884541640654, 2.8188839610583316, 2.3158879734420954, 2.334653328843431, 2.3751365251972985, 2.4238198263324695, 2.4717792647178034, 2.514848566369931, 2.555003951313538, 2.5919002511243088, 2.6257747186158844, 2.653700668896826, 2.6757295847117124, 2.697601649129442, 2.7182867360527414, 2.732479204379476, 2.74471523307909, 2.7533725574405614, 2.7616548966630807, 2.764130363621217, 2.7657590592939294, 2.2900992757661354, 2.3052373411332345, 2.3408120702512694, 2.3863658470930544, 2.4307625657786436, 2.4687541687154013, 2.5062212556052352, 2.541790479530629, 2.5721200886672095, 2.598439369188138, 2.6222284263428426, 2.6427817678884478, 2.659903781761481, 2.6743812861950405, 2.6858800185168428, 2.6941400582634114, 2.700529592833158, 2.7045660651345798, 2.7066081675391604, 2.259235346031739, 2.2708863077094392, 2.30186334529631, 2.3417254197323403, 2.3814274565447313, 2.416271690108693, 2.4506487990414483, 2.484192998500694, 2.512144702967657, 2.536313747021159, 2.558023518859083, 2.5777160943799244, 2.593920022033829, 2.607756027597739, 2.6189430250224723, 2.6270535829437507, 2.6341924724784342, 2.637011577176769, 2.6384940165840556, 2.220210166383371, 2.228604356200259, 2.253701586209948, 2.2880886028809035, 2.3237292296665646, 2.3544433903813884, 2.38588913424697, 2.416157199405339, 2.44208541847349, 2.4640734865814595, 2.483430428747955, 2.5014677538275563, 2.517548269196678, 2.529842321450986, 2.539231719363952, 2.547169766666745, 2.552894533431566, 2.5564004938563545, 2.5579639991190097, 2.170129019475753, 2.1752481019937617, 2.1948604897554085, 2.222290377208274, 2.251402504004785, 2.2785020167160894, 2.305941380612529, 2.331940638563486, 2.355791196616135, 2.3749772752480527, 2.392203878331364, 2.40829440101145, 2.4226408161080473, 2.4343636777940874, 2.442258207625548, 2.4491471702855887, 2.455225474602491, 2.4580452103119077, 2.4595552996241477, 2.1388703075628865, 2.14310994691767, 2.1588467025521054, 2.182750040017008, 2.208820025296224, 2.234098961921123, 2.25739872640121, 2.2813113555610403, 2.302381103829889, 2.3211207830190337, 2.336705235173429, 2.3517208567333325, 2.3637825665278984, 2.3760663951051386, 2.3833188930501366, 2.390259724690552, 2.39516056128754, 2.398243072183643, 2.399198688651199, 2.103106396207975, 2.1055858580074953, 2.1179118773200525, 2.1372275909775755, 2.158688872652917, 2.1788271310352627, 2.199872620246919, 2.222148474330152, 2.240582464543631, 2.2575547029220413, 2.270334086725242, 2.2844236525152906, 2.295734171188186, 2.304734074186056, 2.3129294552874535, 2.319645932508828, 2.3240772720804843, 2.3264876888333275, 2.328934381523818, 2.062672049863547, 2.0603578405384124, 2.068736979722323, 2.079030993167646, 2.096030061752363, 2.1102045261773608, 2.1264836177437187, 2.14560553298252, 2.1600330708935993, 2.1747041296043985, 2.1861316598790252, 2.1971209732448242, 2.2080460882958683, 2.2142151042228972, 2.2263180586584856, 2.22888851584425, 2.2345163014586076, 2.2362468566696942, 2.2372400818313447, 2.008158887869133, 2.0039875824271043, 2.003536094758659, 2.005922505161834, 2.013099244770569, 2.0220456271373544, 2.02944290763973, 2.0401618078465042, 2.050427029760431, 2.0630700092522662, 2.065810154556547, 2.0784776331032386, 2.0860819442264806, 2.0914336463851146, 2.0957559686116736, 2.1017074652566765, 2.1060469717271464, 2.104549297300664, 2.1139565471797277, 1.9575788692332172, 1.9638754448679856, 1.9718851848727175, 1.9657952573738435, 1.9656095922632972, 1.9684471598944637, 1.964530710649968, 1.9630488586900885, 1.9737393912563916, 1.9787210752237252, 1.9950392155024053, 1.9926978447339572, 1.9955596231884831, 2.0001865052800407, 2.0080080426725826, 2.0054975528492105, 2.0000078973718614, 2.0175964547338414, 2.021975623143927], [2.9316284744959002, 2.929881477805574, 2.9257250223026987, 2.917722075662993, 2.907652979284234, 2.894239919140341, 2.877505922398795, 2.8563540026666883, 2.8322389597734614, 2.8051956731962187, 2.7747012472666093, 2.737754462805601, 2.695038473355379, 2.647896167071862, 2.5972697210789715, 2.5451810967499258, 2.483314108891595, 2.429344288341355, 2.4047536835037198, 2.874359544318961, 2.874416718219366, 2.870070938333403, 2.861745975235094, 2.849872128855767, 2.8407023272977865, 2.823445301860041, 2.802007481893269, 2.7795390318909603, 2.7541545449172755, 2.723575023138117, 2.6882208511098544, 2.6502011926536486, 2.6042743447956163, 2.5607784404159464, 2.5085053460411464, 2.4535044878158234, 2.4046965022006166, 2.385074259288955, 2.8120202846450195, 2.8110647501828763, 2.807070737412165, 2.8002834462357233, 2.789430669439989, 2.7791719495193767, 2.7627114786855547, 2.743433676694533, 2.722277554090869, 2.697184461313889, 2.670278751021169, 2.6366281689017925, 2.5985140216684437, 2.5563365634294906, 2.515727783420509, 2.4675550084744655, 2.4168745382417525, 2.3754795919178897, 2.360396685958241, 2.741182649950543, 2.7407401618922655, 2.737515162621723, 2.730616052691592, 2.719946611996146, 2.7104369685913996, 2.6948099367453247, 2.677392775417205, 2.6554016487178655, 2.6324570264792277, 2.6077087089170816, 2.575955939444447, 2.5416134066039042, 2.502892906162658, 2.46598641663544, 2.42164156858856, 2.3773936133675067, 2.3418766992389477, 2.329645594637598, 2.6578836922781353, 2.6566140989136295, 2.652693686630853, 2.646540167561207, 2.6377331025544257, 2.6284150669358177, 2.614653392837992, 2.5984478179293506, 2.5787888873502567, 2.557654563521384, 2.5345096975866337, 2.5063743788185424, 2.4747007316821454, 2.4401875997107205, 2.4064660035973326, 2.3676313057223175, 2.329427806814132, 2.299499484950037, 2.2900290779522594, 2.555615633882789, 2.553933483698276, 2.550899449511171, 2.5445722334409013, 2.5381504130275676, 2.5282010087853983, 2.516047600813006, 2.5009302356624836, 2.484481164372988, 2.465345448092808, 2.4448336972957656, 2.4200098586485472, 2.3922233075293238, 2.3621283582934387, 2.3334807173521246, 2.3006666252684655, 2.2697560352357065, 2.2478443043679976, 2.241585488831333, 2.492740016189521, 2.49231986086783, 2.4887143147054815, 2.48324334784336, 2.475365224081277, 2.46743201986396, 2.4565234278259576, 2.4428068912367107, 2.4267895055529904, 2.410361598342655, 2.391249079129392, 2.368706391590628, 2.3430220401927895, 2.3170506850911354, 2.2906883720483218, 2.262051065297515, 2.2347724676556395, 2.2161551624453124, 2.2115758068653273, 2.4184506588112717, 2.4177188174051123, 2.4148584235364052, 2.4098137791561305, 2.4021899140704828, 2.395061064659339, 2.384310999004003, 2.3734655585315605, 2.3588524311755443, 2.3444593128731412, 2.3263376321193308, 2.3070234980919864, 2.284908680003452, 2.260756790777089, 2.239596052733616, 2.2160846035695516, 2.194216077726144, 2.1800156722641155, 2.1785288618302885, 2.325466714993374, 2.322340734523727, 2.322815193205472, 2.3155822498434677, 2.3114415975864318, 2.3038554567246394, 2.2942966064052577, 2.2861110610925035, 2.272761082213082, 2.2610336823042854, 2.246443793577867, 2.229558447477903, 2.2127115999283027, 2.191902457259438, 2.1801952510387896, 2.1607837959550262, 2.147426327908158, 2.1389030046037796, 2.138911282081512, 2.1976404350378567, 2.194951906209354, 2.192027371675612, 2.187152507801019, 2.1837401331474653, 2.1809144764269583, 2.1722597936161585, 2.165147490497374, 2.156802815974306, 2.1512481057232393, 2.1361673035829787, 2.129298936929126, 2.117873159767733, 2.106163491841994, 2.0962651165977686, 2.0891387266941703, 2.0837032208741397, 2.078691897124856, 2.08608552058544, 2.0993450708002266, 2.108185972339381, 2.1172539074645957, 2.107417189341355, 2.1021547889051, 2.0990573928252814, 2.0859254402479026, 2.0738583707786344, 2.073445342099694, 2.0669094436170874, 2.070834197701101, 2.0566333134353028, 2.0480645848067485, 2.0431501331204016, 2.0425933159008554, 2.0360097778954516, 2.0297592737895616, 2.044171797128649, 2.050467714919871]}]
  out "E1', E2' map coloured by angle set":cluster{dbl[], dbl[]}[](graph)=[{[1.960391667, 1.96395, 1.964858333, 1.964783333, 1.965066667, 1.966358333, 1.967341667, 1.970533333, 1.975933333, 1.981208333, 1.986991667, 1.9887, 1.993983333, 1.998525, 2.003366667, 2.007291667, 2.010375, 2.016083333, 2.018775], [2.103616667, 2.109066667, 2.109416667, 2.105108333, 2.0985, 2.092875, 2.0864, 2.0802, 2.075791667, 2.070616667, 2.065508333, 2.05615, 2.051216667, 2.046983333, 2.04455, 2.042183333, 2.040566667, 2.041175, 2.041491667]}, {[2.003158333, 2.0046, 2.007483333, 2.011925, 2.017033333, 2.023633333, 2.031341667, 2.039791667, 2.048641667, 2.058325, 2.065033333, 2.074866667, 2.0833, 2.091008333, 2.097208333, 2.102025, 2.106216667, 2.108983333, 2.111291667], [2.196025, 2.1949, 2.19305, 2.190366667, 2.185541667, 2.181208333, 2.173725, 2.164375, 2.154508333, 2.145875, 2.134325, 2.124766667, 2.11475, 2.105883333, 2.099075, 2.092341667, 2.087325, 2.083725, 2.081883333]}, {[2.060208333, 2.064741667, 2.072175, 2.081791667, 2.095133333, 2.108266667, 2.1245, 2.142166667, 2.157833333, 2.172066667, 2.185325, 2.197891667, 2.208575, 2.217716667, 2.226233333, 2.229908333, 2.234983333, 2.235541667, 2.236725], [2.323666667, 2.323491667, 2.322275, 2.317708333, 2.312816667, 2.3057, 2.296391667, 2.285258333, 2.271758333, 2.258241667, 2.243808333, 2.226825, 2.208425, 2.191175, 2.177658333, 2.162958333, 2.152308333, 2.143033333, 2.137716667]}, {[2.105091667, 2.111791667, 2.121716667, 2.136008333, 2.154291667, 2.173241667, 2.19535, 2.218758333, 2.2397, 2.256583333, 2.269983333, 2.284675833, 2.2971475, 2.306991667, 2.31468, 2.320805833, 2.324709167, 2.326833333, 2.327125], [2.41685, 2.417708333, 2.415258333, 2.41095, 2.404283333, 2.396708333, 2.38685, 2.374166667, 2.359416667, 2.343625, 2.323891667, 2.303116667, 2.279125, 2.25485, 2.234733333, 2.214875, 2.1991, 2.187875, 2.180358333]}, {[2.143483333, 2.150208333, 2.161633333, 2.179216667, 2.202183333, 2.225733333, 2.251916667, 2.27894, 2.30210675, 2.321888333, 2.337666667, 2.353325, 2.365825, 2.377158333, 2.384858333, 2.390858333, 2.395575, 2.398058333, 2.397933333], [2.4913675, 2.491859167, 2.48918, 2.4840725, 2.477223333, 2.469213333, 2.458326667, 2.445091667, 2.428025, 2.410883333, 2.390291667, 2.365016667, 2.336533333, 2.30825, 2.282841667, 2.258141667, 2.238508333, 2.225533333, 2.217008333]}, {[2.1775, 2.183025, 2.196016667, 2.216541667, 2.243858333, 2.270291667, 2.299676, 2.329216667, 2.355975, 2.376091667, 2.393766667, 2.410083333, 2.424366667, 2.435758333, 2.443616667, 2.450191667, 2.455341667, 2.457883333, 2.4582], [2.55425, 2.553541667, 2.551325, 2.545416667, 2.538966667, 2.53025, 2.518325, 2.503135833, 2.486316667, 2.466695, 2.444466667, 2.41635, 2.385666667, 2.352891667, 2.323591667, 2.294933333, 2.272216667, 2.257616667, 2.24995]}, {[2.232116667, 2.237608333, 2.252575, 2.280024167, 2.3128225, 2.345008333, 2.379466667, 2.413575, 2.442833333, 2.466116667, 2.48555, 2.503733333, 2.519275, 2.53135, 2.54055, 2.548033333, 2.553266667, 2.555883333, 2.556633333], [2.6561, 2.656033333, 2.653025, 2.6479, 2.6395, 2.630575, 2.617266667, 2.601025, 2.581183333, 2.559808333, 2.534183333, 2.502759167, 2.4664025, 2.428383333, 2.393575, 2.357791667, 2.328641667, 2.31185, 2.30585]}, {[2.274035, 2.2802375, 2.299259333, 2.332033333, 2.369858333, 2.406766667, 2.444191667, 2.481825, 2.51305, 2.53835, 2.560558333, 2.579975, 2.596066667, 2.609508333, 2.619975, 2.627683333, 2.63435, 2.636566667, 2.637225], [2.73945, 2.740158333, 2.737916667, 2.731575, 2.721716667, 2.712475, 2.697358333, 2.680066667, 2.658041667, 2.635133333, 2.608125, 2.573008333, 2.533166667, 2.490545, 2.451891667, 2.409791667, 2.374775, 2.354208333, 2.349541667]}, {[2.307579167, 2.314378333, 2.337491667, 2.375958333, 2.418925, 2.4591, 2.499458333, 2.539283333, 2.573725, 2.600716667, 2.624725, 2.6453, 2.661966667, 2.67585, 2.686825, 2.694791667, 2.700691667, 2.704191667, 2.705316667], [2.810258333, 2.8105, 2.807475, 2.801341667, 2.7911, 2.781116667, 2.765166667, 2.746433333, 2.724641667, 2.699766667, 2.671158333, 2.633491667, 2.590441667, 2.544425, 2.501685, 2.45417, 2.412591667, 2.3881, 2.383508333]}, {[2.334358333, 2.3435, 2.371475, 2.414241667, 2.460875, 2.50545, 2.548441667, 2.589525, 2.626741667, 2.655541667, 2.678608333, 2.700075, 2.72025, 2.733825, 2.745575, 2.754075, 2.761891667, 2.763625, 2.764575], [2.872791667, 2.873891667, 2.870325, 2.862483333, 2.8512, 2.8425, 2.825866667, 2.804941667, 2.78255, 2.757241667, 2.724783333, 2.685333333, 2.642233333, 2.592433333, 2.546675, 2.494478333, 2.447691667, 2.417191667, 2.41095]}, {[2.357966667, 2.367716667, 2.400833333, 2.449375, 2.501233333, 2.545475, 2.591691667, 2.635783333, 2.674008333, 2.703908333, 2.729233333, 2.752258333, 2.77055, 2.786458333, 2.796925, 2.807291667, 2.813483333, 2.817483333, 2.817816667], [2.929983333, 2.929458333, 2.92605, 2.918566667, 2.908825, 2.896141667, 2.879666667, 2.859191667, 2.835225, 2.808475, 2.775591667, 2.734741667, 2.686808333, 2.635733333, 2.585316667, 2.530825, 2.476695, 2.441908333, 2.433175]}]
  out "Probe angles traversed in each angle set\n1st index: angle (deg)\n2nd index: angle set":dbl[][](array[numeric])=[[-45.0, -45.0, -45.0, -45.0, -45.0, -45.0, -45.0, -45.0, -45.0, -45.0, -45.0], [-40.23, -40.23, -40.23, -40.23, -40.23, -40.23, -40.23, -40.23, -40.14, -40.14, -40.14], [-35.1, -35.1, -35.1, -35.1, -35.1, -35.1, -35.1, -35.1, -35.1, -35.1, -35.1], [-29.88, -29.88, -29.88, -29.88, -29.88, -29.88, -29.88, -29.88, -29.88, -29.97, -29.88], [-24.75, -24.75, -24.75, -24.75, -24.75, -25.02, -24.75, -24.75, -24.75, -24.84, -24.84], [-20.25, -20.25, -20.25, -20.25, -19.98, -20.25, -20.25, -20.25, -20.25, -20.25, -20.25], [-15.21, -15.21, -15.21, -15.21, -15.21, -15.21, -15.21, -15.21, -15.21, -15.21, -15.21], [-9.99, -9.99, -9.99, -9.99, -9.99, -9.99, -9.99, -9.99, -9.99, -9.99, -9.99], [-4.86, -4.86, -4.86, -4.86, -4.86, -4.86, -4.86, -4.86, -5.04, -4.86, -4.86], [0.0, 0.0, 0.0, 0.0, 0.0, 0.0, 0.0, 0.0, -0.09, 0.0, 0.0], [4.77, 4.77, 4.77, 4.77, 4.77, 4.77, 4.77, 4.77, 4.77, 4.77, 4.77], [9.9, 9.9, 9.9, 9.9, 9.9, 9.9, 9.9, 9.99, 9.9, 9.9, 9.9], [15.12, 15.12, 15.03, 15.03, 15.03, 15.12, 15.12, 15.03, 15.03, 15.03, 15.03], [19.98, 20.16, 20.25, 20.16, 20.16, 20.25, 20.16, 20.16, 20.16, 20.16, 20.16], [24.84, 24.84, 24.75, 24.75, 24.75, 24.75, 24.75, 24.75, 24.75, 24.75, 25.02], [29.79, 29.79, 29.79, 29.79, 29.79, 29.79, 29.79, 29.79, 29.7, 29.7, 29.7], [35.01, 35.01, 35.01, 35.01, 35.01, 35.01, 34.92, 35.01, 34.92, 34.92, 34.92], [40.14, 40.14, 40.14, 40.14, 40.14, 39.96, 40.14, 40.14, 40.14, 40.14, 40.14], [45.0, 45.0, 45.0, 45.0, 45.0, 45.0, 45.0, 45.0, 45.0, 45.0, 45.0]]
  out "Uref associated with each angle set (m/s)":dbl[](array[numeric])=[0.5018157894736842, 0.9994315789473684, 2.000205263157895, 3.000784210526316, 3.999947368421053, 4.999831578947369, 6.999731578947368, 9.001931578947369, 10.999973684210525, 13.000168421052631, 15.001142105263158] format="%#.2f"
  out "Zero angle calibration coeffs. (King's 1914 law)":T1={"A1"=2.895294801714706, "B1"=1.359762188126494, "n1"=0.4357683216387929, "A2"=3.2944413738572145, "B2"=1.3280301230872396, "n2"=0.4590330236259289}
  in  "Query set":i32=3
  out "Pts per set":i32=19
  out "Angle sets":i32=11
  # "This vi allows you to inspect the finer details of your angle calibration. You can check the extent of validity of the effective angle method. The probe zero angle alignment error is given graphically, you can then correct the recorded angles in the calibration file by ADDING the value obtained from the graph where the curve has levelled off (which typically occurs at speed > 4m/s. Similarly the effective angle typically becomes constant at speed > 4m/s)."
  # "of"
  # "Paul Nathan 23/02/10"
  # "HIGHER ORDER METHOD\nBELOW"
  # "HIGHER ORDER METHOD\nBELOW"
  # "HIGHER ORDER METHOD\nBELOW"
  # "0. Actual data\n1. Higher order effective angle method\n    with tangential cooling factor"
  # "ADVANCED DIAGNOSTICS: This section reveals the guts of the quartic equation for epsilon and whether the algorithm fell back to the lower order method. You can check all the roots for each angle set and see the effects of constraining the polynomial coefficients (in particular setting the zero order coeff to zero). Since the constraint affects the master plots, be sure to empty the coefficient constraint array when finished."
  # "The numerical data for all the higher order effective angle method plots is available for copying and pasting into Excel below"
  # "The numerical data for the E1, E2 plane maps (actual data, and synthesis from both effective angle methods) is available for copying and pasting into Excel below"
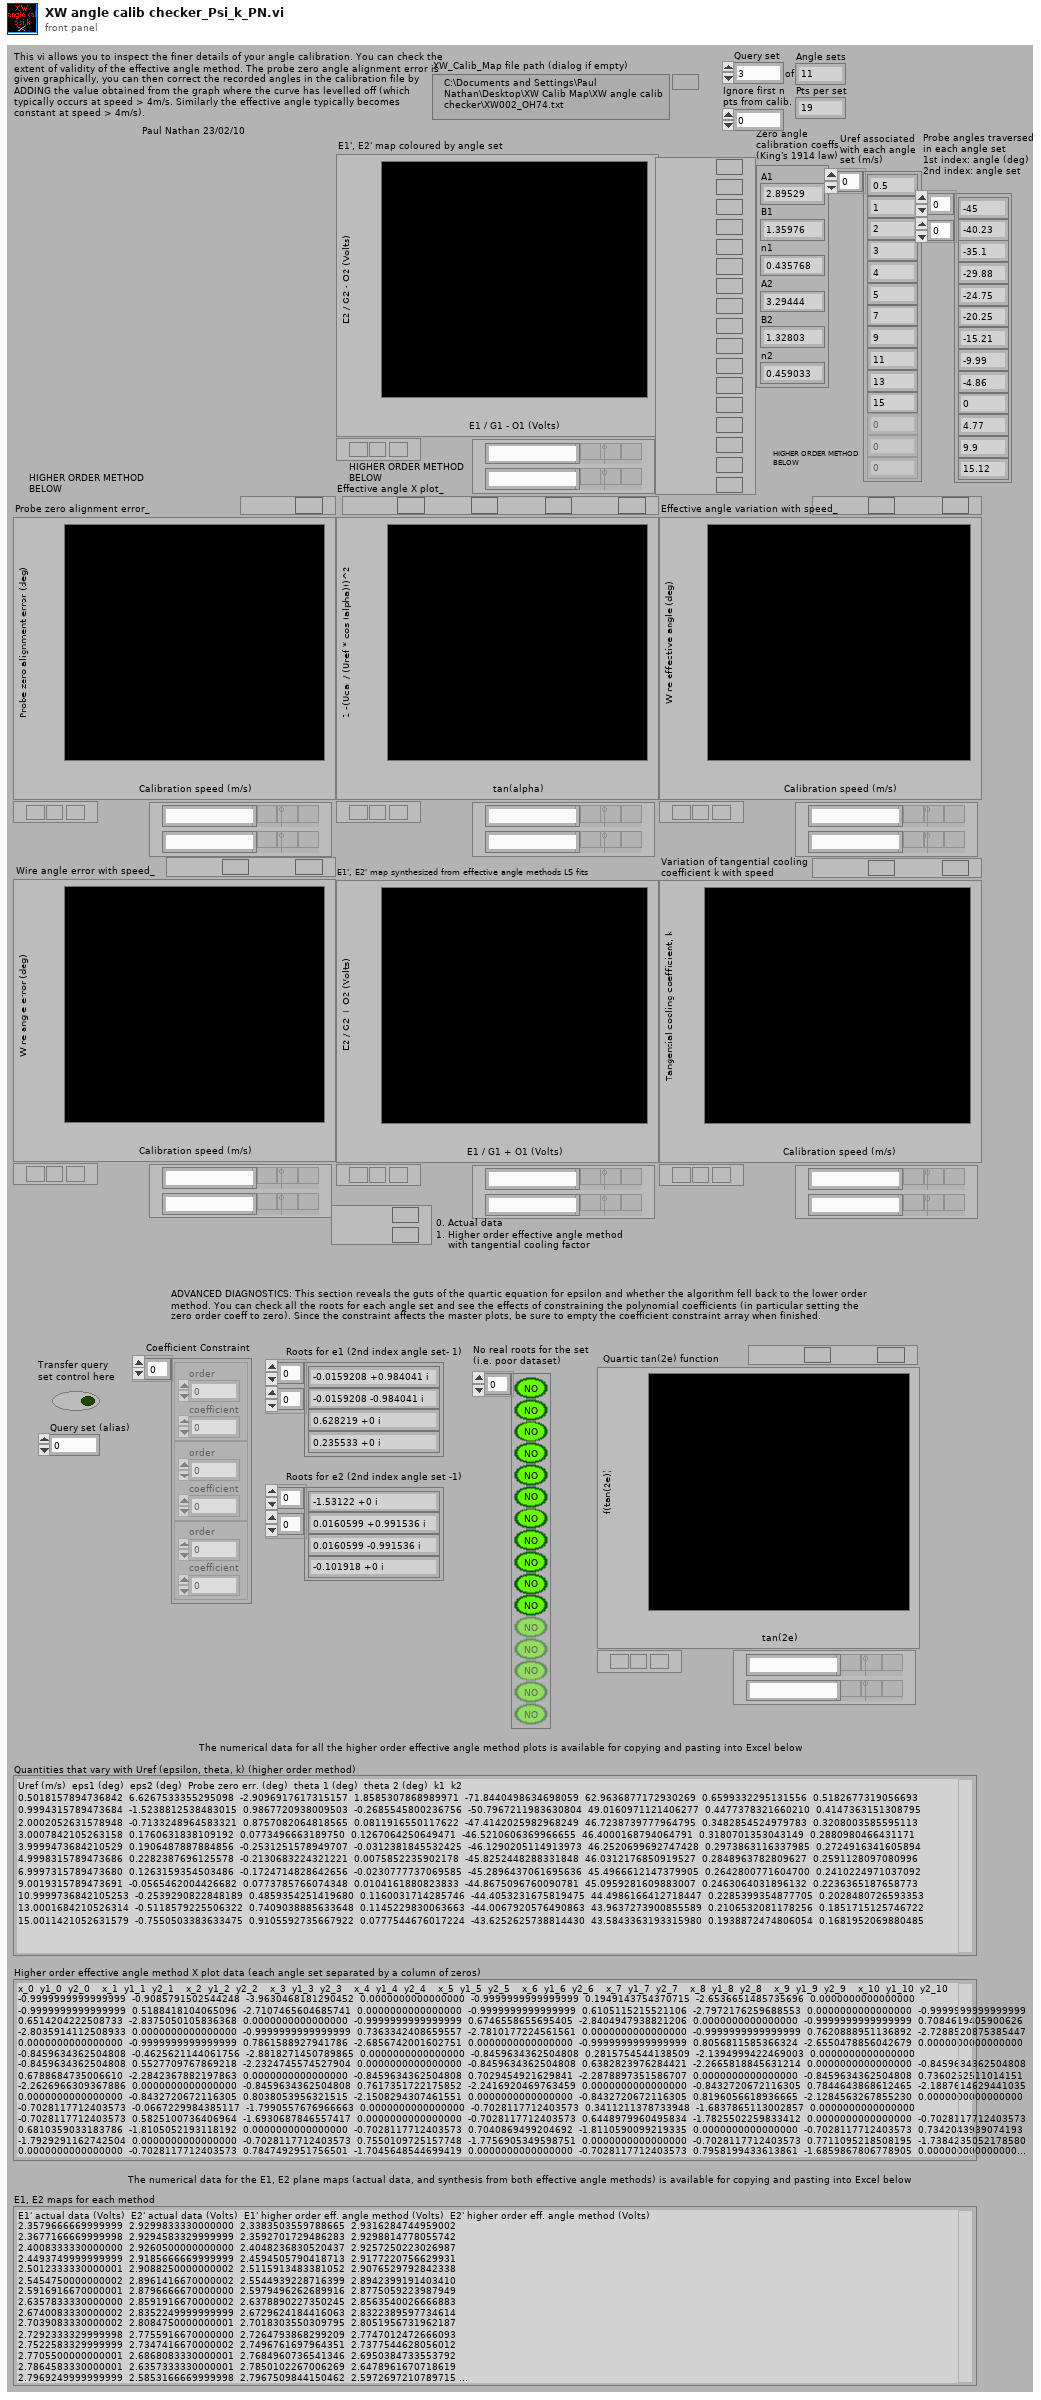
[diagram p1: front panel]
types:
  T1 = cluster{"A1":dbl, "B1":dbl, "n1":dbl, "A2":dbl, "B2":dbl, "n2":dbl}
  T2 = cluster{"A":dbl, "B":dbl, "n":dbl, "A":dbl, "B":dbl, "n":dbl}
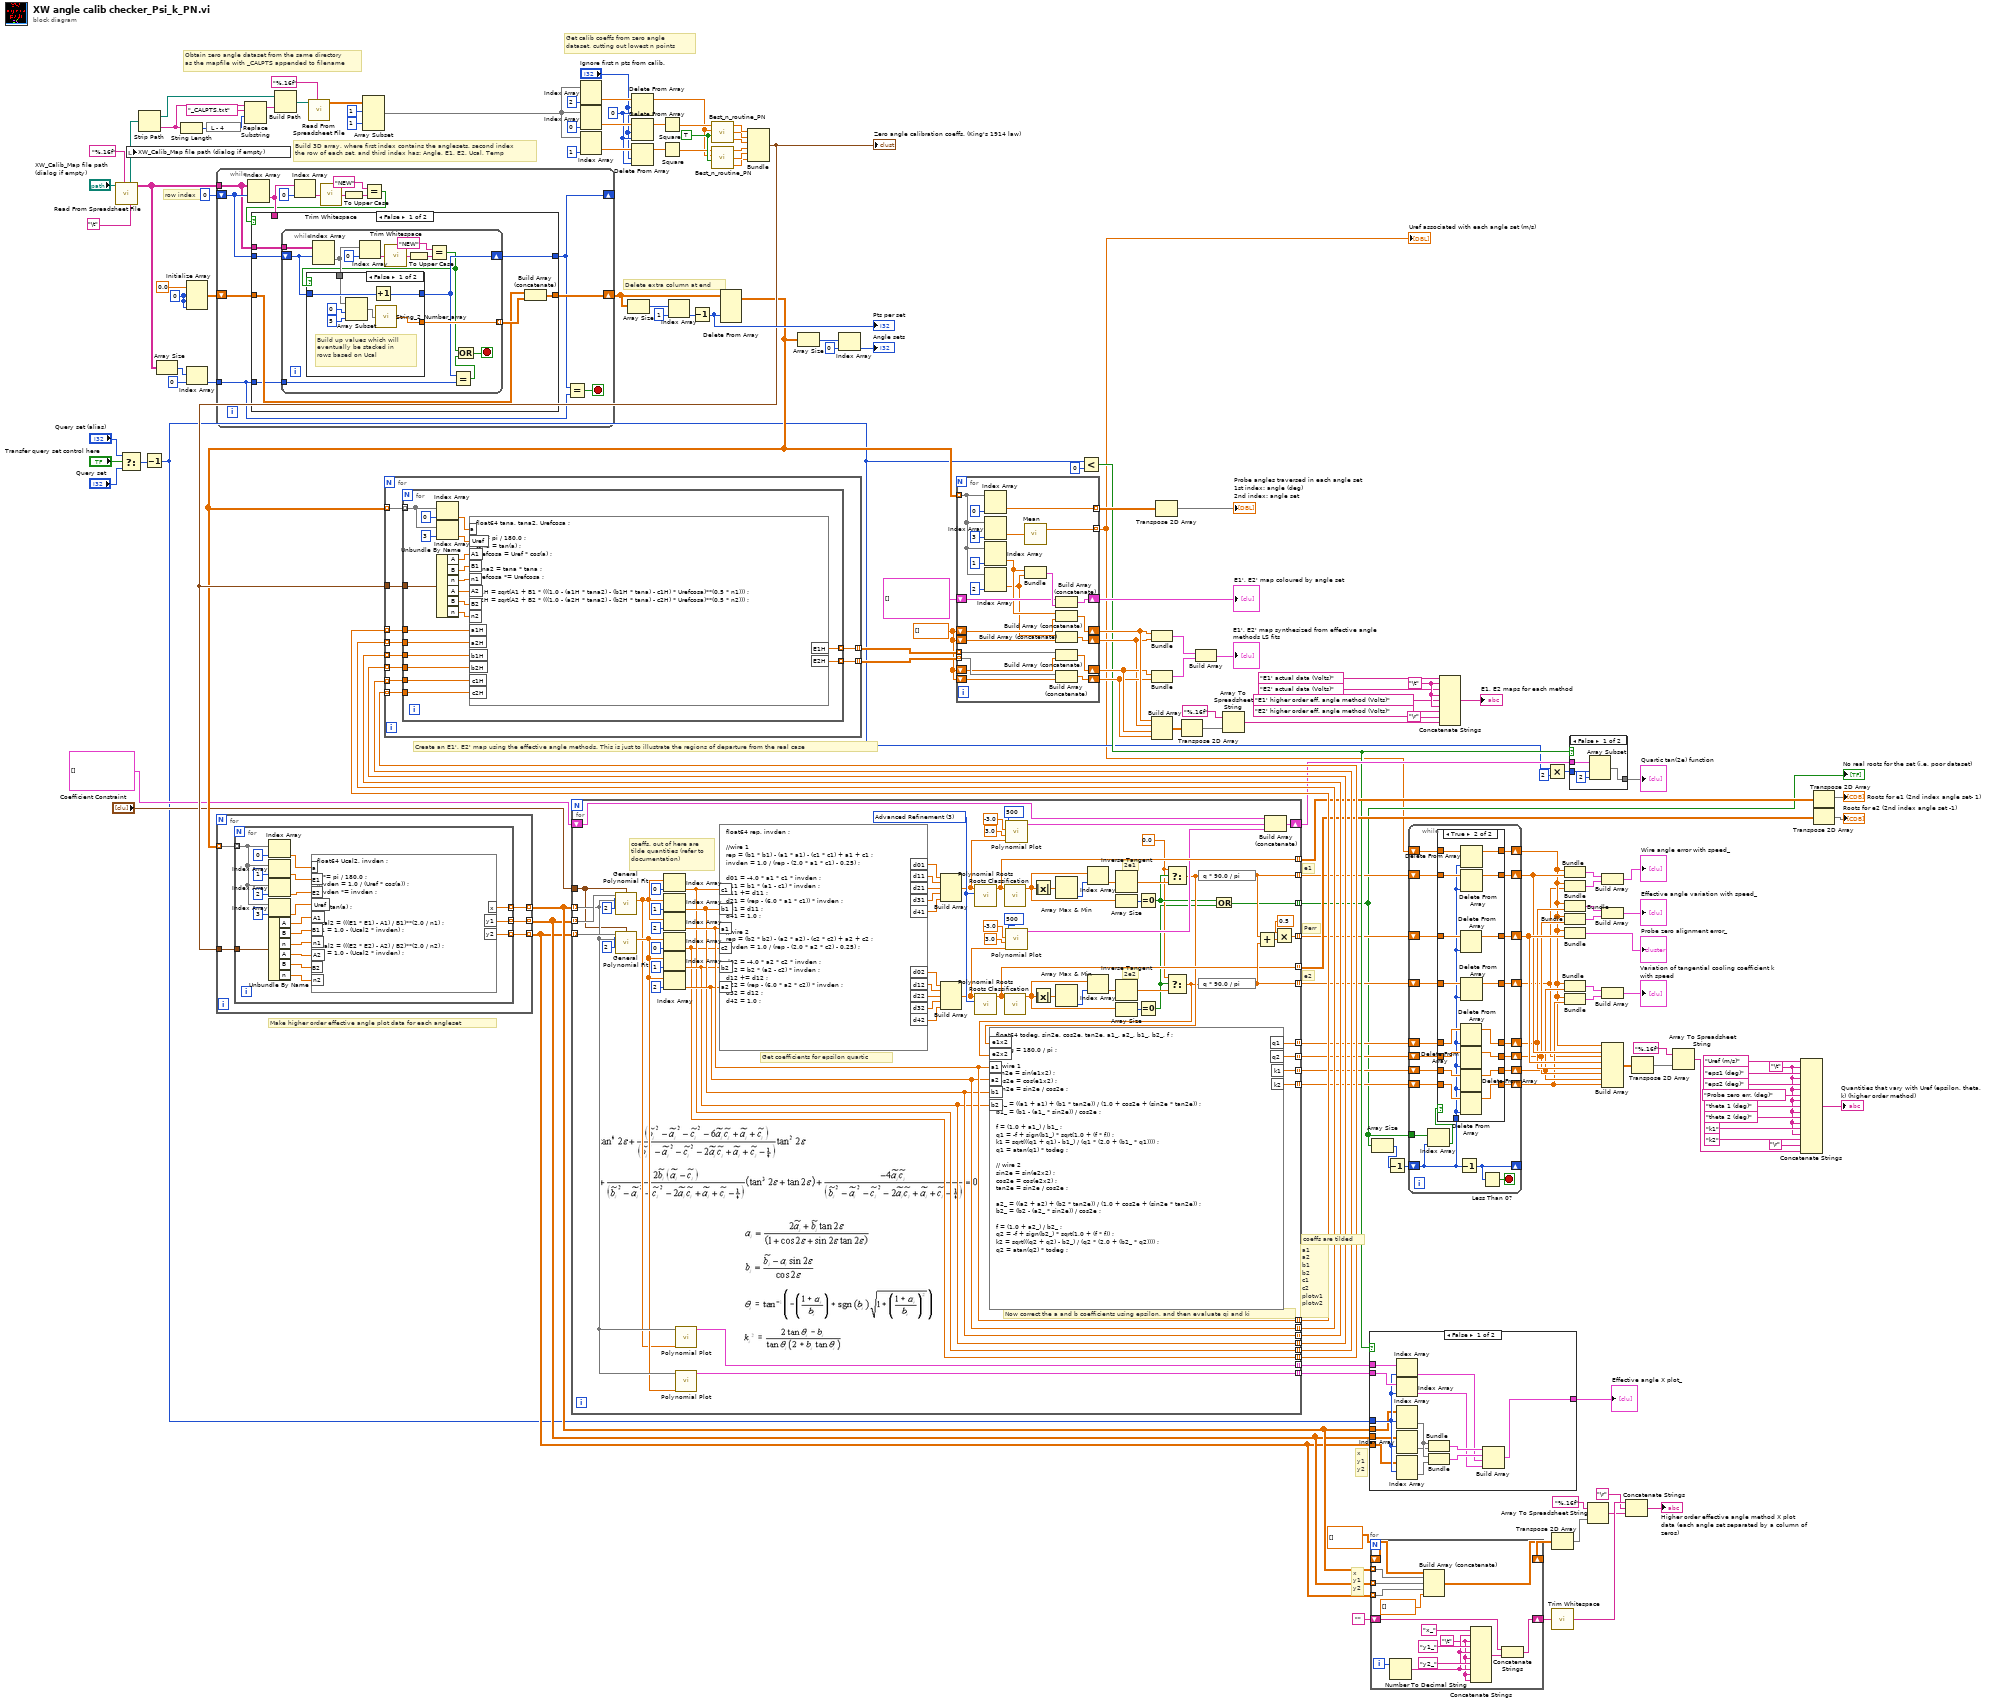
[diagram p0: block diagram]
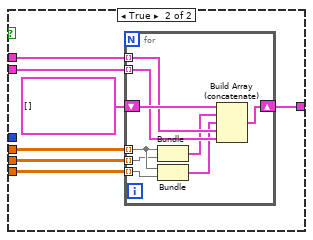
[diagram p4: hidden frame]
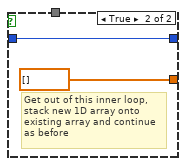
[diagram p5: hidden frame]
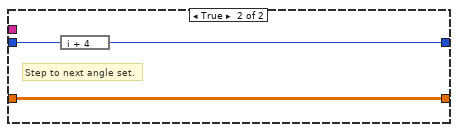
[diagram p6: hidden frame]
diagram:
  w41 = 0 ("index")
  w67 = "\t"
  w78 = "\t"
  w45 = dbl[] []
  w129 = TRUE ("variable n?")
  w146 = 0 ("dimension size")
  # "x\ny1\ny2"
  # "x\ny1\ny2"
  # "coeffs are tilded"
  # "a1\na2\nb1\nb2\nc1\nc2\nplotw1\nplotw2"
  # "Make higher order effective angle plot data for each angleset"
  # "e2"
  # "e1"
  # "Perr"
  # "Create an E1', E2' map using the effective angle methods. This is just to illustrate the regions of departure from the real case"
  # "Get calib coeffs from zero angle dataset, cutting out lowest n points"
  # "Obtain zero angle dataset from the same directory as the mapfile with _CALPTS appended to filename"
  # "Delete extra column at end"
  # "Build 3D array, where first index contains the anglesets, second index the row of each set, and third index has: Angle, E1, E2, Ucal, Temp"
  # "row index"
  n1 = call-poly <vilib>:"Read From Spreadsheet File.vi"("delimiter (\\t)"="\t", "format (%s)"="%.16f" ("format (%.3f)"), "file path (dialog if empty)"="XW_Calib_Map file path (dialog if empty)") -> ("all rows"=w160:string[][], "new file path (Not A Path if cancelled)"=w132:path)  [unwired: 2 in, 5 out]
  n2 = Select(t="Query set (alias)", s="Transfer query set control here", f="Query set") -> (s? t:f=w24:i32)
  n3 = local write "XW_Calib_Map file path (dialog if empty)"(w132) -> ()
  n4 = Strip Path(path=w132) -> (stripped path=w139:path, name=w143:string)
  n5 = Decrement(x=w24) -> (x-1=w22:i32)
  n6 = Array Size(array=w160) -> (size(s)=w157:i32[])
  n7 = String Length(string=w143) -> (length=w142:i32)
  n8 = Initialize Array(0.0 ("element"), w146, w146, w146) -> (w145:dbl[][][])
  n9 = Index Array(array=w157, index=0) -> (element=w156:i32)
  n10 = expression code="L - 4"(w142) -> (w141:i32)
  n11 = while {
    tunnel: w160 -> [w169]
    shift-right: [w167] -> w150
    shift-left: w145 -> [w168]
    shift-right: [w166] -> _
    shift-left: 0 ("index") -> [w172]
    tunnel: w156 -> [w165]
    stop <- w174 stop-if-true
    n12 = Index Array(array=w169, index (row)=w172) -> (element=w171:string[])  [unwired: 1 in]
    n13 = Index Array(array=w171, index=0) -> (element=w164:string)
    n14 = call <vilib>:"Trim Whitespace.vi"("string"=w164) -> ("trimmed string"=w163:string)  [unwired: 1 in]
    n15 = To Upper Case(1:w163) -> (0:w176:string)
    n16 = Equal?(x="NEW", y=w176) -> (x = y?=w170:bool)
    n17 = case shown="False" w170 {
      tunnel: w172 -> [w183 w209]
      tunnel: [w178 w207] -> w166
      tunnel: w171 -> [_ _]
      tunnel: w169 -> [w182 _]
      tunnel: w168 -> [w179 w208]
      tunnel: [w181 w208] -> w167
      tunnel: w165 -> [w177 _]
      frame False {
        n18 = while {
          tunnel: w182 -> [w193]
          shift-right: [w188] -> w178
          shift-left: w183 -> [w191]
          tunnel: [w192] -> w180 mode=indexing
          tunnel: w177 -> [w190]
          stop <- w187 stop-if-true
          n19 = Index Array(array=w193, index (row)=w191) -> (element=w194:string[])  [unwired: 1 in]
          n20 = Index Array(array=w194, index=0) -> (element=w185:string)
          n21 = call <vilib>:"Trim Whitespace.vi"("string"=w185) -> ("trimmed string"=w184:string)  [unwired: 1 in]
          n22 = To Upper Case(1:w184) -> (0:w197:string)
          n23 = Equal?(x="NEW", y=w197) -> (x = y?=w186:bool)
          n24 = case shown="False" w186 {
            tunnel: w194 -> [w199 _]
            tunnel: [w198 dbl[] []] -> w192
            tunnel: w191 -> [w202 w206]
            tunnel: [w201 w206] -> w188
            frame False {
              # "Build up values which will eventually be stacked in rows based on Ucal"
              n25 = Array Subset(array=w199, index=0, length=5) -> (w203:string[])
              n26 = Increment(x=w202) -> (x+1=w201:i32)
              n27 = call "String_2_Number_array.vi"("Input String"=w203) -> ("Values"=w198:dbl[])
            }
            frame True {
              # "Get out of this inner loop, stack new 1D array onto existing array and continue as before"
            }
          }
          n28 = Equal?(x=w188, y=w190) -> (x = y?=w189:bool)
          n29 = Or(x=w186, y=w189) -> (x .or. y?=w187:bool)
        }
        n30 = Build Array (concatenate)(w179, w180) -> (w181:dbl[][][])
      }
      frame True {
        # "Step to next angle set."
        n31 = expression code="i + 4"(w209) -> (w207:i32)
      }
    }
    n32 = Equal?(x=w166, y=w165) -> (x = y?=w174:bool)
  }
  n33 = Replace Substring(3:w141, 4:"_CALPTS.txt" ("substring (\"\")"), 5:w143) -> (1:w138:string)  [unwired: 2 out]
  n34 = Build Path(base path=w139, name or relative path=w138) -> (appended path=w133:path)
  n35 = call-poly <vilib>:"Read From Spreadsheet File.vi"("format (%.3f)"="%.16f", "file path (dialog if empty)"=w133) -> ("all rows"=w135:dbl[][])  [unwired: 2 in, 7 out]
  n36 = Array Subset(array=w135, index (row)=1 ("index"), index (col)=1 ("index")) -> (w130:dbl[][])  [unwired: 2 in]
  n37 = Index Array(array=w130, index (col)=2 ("index")) -> (element=w44:dbl[])  [unwired: 1 in]
  n38 = Index Array(array=w130, index (col)=0 ("index")) -> (element=w43:dbl[])  [unwired: 1 in]
  n39 = Index Array(array=w130, index (col)=1 ("index")) -> (element=w42:dbl[])  [unwired: 1 in]
  n40 = Array Size(array=w150) -> (size(s)=w152:i32[])
  n41 = Delete From Array(array=w44, length="Ignore first n pts from calib.", index=w41) -> (array with subset deleted=w40:dbl[])  [unwired: 1 out]
  n42 = Delete From Array(array=w43, length="Ignore first n pts from calib.", index=w41) -> (array with subset deleted=w39:dbl[])  [unwired: 1 out]
  n43 = Delete From Array(array=w42, length="Ignore first n pts from calib.", index=w41) -> (array with subset deleted=w38:dbl[])  [unwired: 1 out]
  n44 = Square(x=w39) -> (x^2=w120:dbl[])
  n45 = Square(x=w38) -> (x^2=w119:dbl[])
  n46 = Index Array(array=w152, index=1) -> (element=w151:i32)
  n47 = Decrement(x=w151) -> (x-1=w148:i32)
  "Pts per set" <- w148
  n48 = call "Best_n_routine_PN.vi"("variable n?"=w129, "U"=w40, "E^2"=w120) -> ("n"=w124:dbl, "B"=w125:dbl, "A"=w126:dbl)  [unwired: 1 in]
  n49 = call "Best_n_routine_PN.vi"("variable n?"=w129, "U"=w40, "E^2"=w119) -> ("n"=w121:dbl, "B"=w122:dbl, "A"=w123:dbl)  [unwired: 1 in]
  n50 = Delete From Array(array=w150, index (dim 1)=w148) -> (array with subset deleted=w110:dbl[][][])  [unwired: 3 in, 1 out]
  n51 = Bundle("A"=w126, "B"=w125, "n"=w124, "A"=w123, "B"=w122, "n"=w121) -> (w111:T2)  [unwired: 1 out]
  "Zero angle calibration coeffs. (King's 1914 law)" <- w111
  n52 = for {
    tunnel: w110 -> [w214] mode=indexing
    tunnel: w111 -> [w213]
    tunnel: [w212] -> w49 mode=indexing
    tunnel: [w211] -> w48 mode=indexing
    tunnel: [w210] -> w47 mode=indexing
    n53 = for {
      tunnel: w214 -> [w219] mode=indexing
      tunnel: w213 -> [w232]
      tunnel: [w217] -> w212 mode=indexing
      tunnel: [w216] -> w211 mode=indexing
      tunnel: [w215] -> w210 mode=indexing
      n54 = Index Array(array=w219, index=0) -> (element=w231:dbl)
      n55 = Index Array(array=w219, index=1) -> (element=w220:dbl)
      n56 = Index Array(array=w219, index=2) -> (element=w218:dbl)
      n57 = Index Array(array=w219, index=3) -> (element=w221:dbl)
      n58 = Unbundle By Name(w232) -> ("A"=w230:dbl, "B"=w229:dbl, "n"=w228:dbl, "A"=w227:dbl, "B"=w226:dbl, "n"=w225:dbl)
      n59 = formula code="float64 Ucal2, invden ;\n\na *= pi / 180.0 ;\ninvden = 1.0 / (Uref * cos(a)) ;\ninvden *= invden ;\n\nx = tan(a) ;\n\nUcal2 = (((E1 * E1) - A1) / B1)**(2.0 / n1) ;\ny1 = 1.0 - (Ucal2 * invden) ;\n\nUcal2 = (((E2 * E2) - A2) / B2)**(2.0 / n2) ;\ny2 = 1.0 - (Ucal2 * invden) ;"("A1"=w230, "B1"=w229, "n1"=w228, "A2"=w227, "B2"=w226, "n2"=w225, "E1"=w220, "E2"=w218, "a"=w231, "Uref"=w221) -> ("x"=w217:dbl, "y1"=w216:dbl, "y2"=w215:dbl)
    }
  }
  n60 = for {
    tunnel: w49 -> [w277] mode=indexing
    tunnel: w48 -> [w306] mode=indexing
    tunnel: w47 -> [w298] mode=indexing
    tunnel: [w278] -> w19 mode=indexing
    tunnel: [w276] -> w20 mode=indexing
    tunnel: [w275] -> w18 mode=indexing
    tunnel: [w274] -> w17 mode=indexing
    tunnel: [w273] -> w16 mode=indexing
    tunnel: [w272] -> w15 mode=indexing
    tunnel: [w271] -> w14 mode=indexing
    tunnel: [w270] -> w89 mode=indexing
    tunnel: [w269] -> w88 mode=indexing
    tunnel: [w268] -> w109 mode=indexing
    tunnel: [w267] -> w108 mode=indexing
    tunnel: [w266] -> w107 mode=indexing
    tunnel: [w265] -> w106 mode=indexing
    tunnel: [w264] -> w105 mode=indexing
    tunnel: [w263] -> w104 mode=indexing
    tunnel: "Coefficient Constraint" -> [w256]
    tunnel: [w255] -> w35 mode=indexing
    shift-right: [w247] -> w30
    shift-left: cluster{dbl[], dbl[]}[] [] -> [w250]
    tunnel: [w246] -> w32 mode=indexing
    tunnel: [w240] -> w2 mode=indexing
    w239 = 0.0 ("end")
    w287 = u16 3 items=["General", "Simple Classification", "Refinement", "Advanced Refinement"] ("option")
    # "Now correct the a and b coefficients using epsilon, and then evaluate qi and ki"
    # "2e2"
    # "2e1"
    # "coeffs. out of here are tilde quantities (refer to documentation)"
    # "Get coefficients for epsilon quartic"
    n61 = call <vilib>:"General Polynomial Fit.vi"("Y"=w306, "polynomial order"=2, "Coefficient Constraint"=w256, "X"=w277) -> ("Polynomial Coefficients"=w261:dbl[])  [unwired: 8 in, 3 out]
    n62 = call <vilib>:"General Polynomial Fit.vi"("Y"=w298, "polynomial order"=2, "Coefficient Constraint"=w256, "X"=w277) -> ("Polynomial Coefficients"=w262:dbl[])  [unwired: 8 in, 3 out]
    n63 = Index Array(array=w261, index=0) -> (element=w264:dbl)
    n64 = Index Array(array=w261, index=1) -> (element=w266:dbl)
    n65 = Index Array(array=w261, index=2) -> (element=w268:dbl)
    n66 = Index Array(array=w262, index=0) -> (element=w263:dbl)
    n67 = Index Array(array=w262, index=1) -> (element=w265:dbl)
    n68 = Index Array(array=w262, index=2) -> (element=w267:dbl)
    n69 = call-poly <vilib>:"Polynomial Plot.vi"("P(x)"=w261, "X"=w277) -> ("polynomial plot"=w270:cluster{dbl[], "P(A)":dbl[]})  [unwired: 9 out]
    n70 = call-poly <vilib>:"Polynomial Plot.vi"("P(x)"=w262, "X"=w277) -> ("polynomial plot"=w269:cluster{dbl[], "P(A)":dbl[]})  [unwired: 9 out]
    n71 = formula code="float64 rep, invden ;\n\n//wire 1\nrep = (b1 * b1) - (a1 * a1) - (c1 * c1) + a1 + c1 ;\ninvden = 1.0 / (rep - (2.0 * a1 * c1) - 0.25) ;\n\nd01 = -4.0 * a1 * c1 * invden ;\nd11 = b1 * (a1 - c1) * invden ; \nd11 += d11 ;\nd21 = (rep - (6.0 * a1 * c1)) * invden ;\nd31 = d11 ;\nd41 = 1.0 ;\n\n//wire 2\nrep = (b2 * b2) - (a2 * a2) - (c2 * c2) + a2 + c2 ;\ninvden = 1.0 / (rep - (2.0 * a2 * c2) - 0.25) ;\n\nd02 = -4.0 * a2 * c2 * invden ;\nd12 = b2 * (a2 - c2) * invden ;\nd12 += d12 ;\nd22 = (rep - (6.0 * a2 * c2)) * invden ;\nd32 = d12 ;\nd42 = 1.0 ;"("c1"=w264, "a1"=w268, "b1"=w266, "c2"=w263, "b2"=w265, "a2"=w267) -> ("d01"=w297:dbl, "d11"=w296:dbl, "d21"=w295:dbl, "d02"=w290:dbl, "d12"=w291:dbl, "d22"=w292:dbl, "d31"=w294:dbl, "d41"=w293:dbl, "d32"=w289:dbl, "d42"=w288:dbl)
    n72 = Build Array(w297, w296, w295, w294, w293) -> (w260:dbl[])
    n73 = Build Array(w290, w291, w292, w289, w288) -> (w251:dbl[])
    n74 = call-poly <vilib>:"Polynomial Roots.vi"("option"=w287, "P(x)"=w260) -> ("Roots"=w255:cdb[])  [unwired: 9 out]
    n75 = call-poly <vilib>:"Polynomial Roots.vi"("option"=w287, "P(x)"=w251) -> ("Roots"=w246:cdb[])  [unwired: 9 out]
    n76 = call <vilib>:"Roots Classification.vi"("Roots"=w255) -> ("Real Roots"=w237:dbl[])  [unwired: 2 in, 8 out]
    n77 = call <vilib>:"Roots Classification.vi"("Roots"=w246) -> ("Real Roots"=w234:dbl[])  [unwired: 2 in, 8 out]
    n78 = call-poly <vilib>:"Polynomial Plot.vi"("P(x)"=w260, "end"=3.0, "start"=-3.0, "samples"=500) -> ("polynomial plot"=w249:cluster{"Ramp Pattern":dbl[], "P(A)":dbl[]})  [unwired: 7 out]
    n79 = call-poly <vilib>:"Polynomial Plot.vi"("P(x)"=w251, "end"=3.0, "start"=-3.0, "samples"=500) -> ("polynomial plot"=w248:cluster{"Ramp Pattern":dbl[], "P(A)":dbl[]})  [unwired: 7 out]
    n80 = Absolute Value(x=w237) -> (abs(x)=w286:dbl[])
    n81 = Absolute Value(x=w234) -> (abs(x)=w283:dbl[])
    n82 = Array Max & Min(array=w286) -> (min index (indices)=w285:i32)  [unwired: 3 out]
    n83 = Array Max & Min(array=w283) -> (min index (indices)=w284:i32)  [unwired: 3 out]
    n84 = Index Array(array=w237, index=w285) -> (element=w282:dbl)
    n85 = Index Array(array=w234, index=w284) -> (element=w281:dbl)
    n86 = Inverse Tangent(1:w282) -> (0:w245:dbl)
    n87 = Array Size(array=w237) -> (size(s)=w238:i32)
    n88 = Inverse Tangent(1:w281) -> (0:w243:dbl)
    n89 = Array Size(array=w234) -> (size(s)=w236:i32)
    n90 = Equal To 0?(x=w238) -> (x = 0?=w241:bool)
    n91 = Equal To 0?(x=w236) -> (x = 0?=w235:bool)
    n92 = Select(t=w239, s=w241, f=w245) -> (s? t:f=w244:dbl)
    n93 = Select(t=w239, s=w235, f=w243) -> (s? t:f=w242:dbl)
    n94 = formula code="float64 todeg, sin2e, cos2e, tan2e, a1_, a2_, b1_, b2_, f ;\n\ntodeg = 180.0 / pi ;\n\n// wire 1\nsin2e = sin(e1x2) ; \ncos2e = cos(e1x2) ; \ntan2e = sin2e / cos2e ;\n\na1_ = ((a1 + a1) + (b1 * tan2e)) / (1.0 + cos2e + (sin2e * tan2e)) ;\nb1_ = (b1 - (a1_ * sin2e)) / cos2e ;\n\nf = (1.0 + a1_) / b1_ ;\nq1 = -f + sign(b1_) * sqrt(1.0 + (f * f)) ;\nk1 = sqrt(((q1 + q1) - b1_) / (q1 * (2.0 + (b1_ * q1)))) ;\nq1 = atan(q1) * todeg ;\n\n// wire 2\nsin2e = sin(e2x2) ; \ncos2e = cos(e2x2) ; \ntan2e = sin2e / cos2e ;\n\na2_ = ((a2 + a2) + (b2 * tan2e)) / (1.0 + cos2e + (sin2e * tan2e)) ;\nb2_ = (b2 - (a2_ * sin2e)) / cos2e ;\n\nf = (1.0 + a2_) / b2_ ;\nq2 = -f + sign(b2_) * sqrt(1.0 + (f * f)) ;\nk2 = sqrt(((q2 + q2) - b2_) / (q2 * (2.0 + (b2_ * q2)))) ;\nq2 = atan(q2) * todeg ;"("e1x2"=w244, "e2x2"=w242, "a1"=w268, "a2"=w267, "b1"=w266, "b2"=w265) -> ("q1"=w274:dbl, "q2"=w273:dbl, "k1"=w272:dbl, "k2"=w271:dbl)
    n95 = expression code="q * 90.0 / pi"(w244) -> (w276:dbl)
    n96 = expression code="q * 90.0 / pi"(w242) -> (w275:dbl)
    n97 = Or(x=w241, y=w235) -> (x .or. y?=w240:bool)
    n98 = Add(x=w276, y=w275) -> (x+y=w279:dbl)
    n99 = Build Array (concatenate)(w250, w249, w248) -> (w247:cluster{"Ramp Pattern":dbl[], "P(A)":dbl[]}[])
    n100 = Multiply(x=0.5, y=w279) -> (x*y=w278:dbl)
  }
  "No real roots for the set (i.e. poor dataset)" <- w2
  n101 = for {
    tunnel: w110 -> [w317] mode=indexing
    tunnel: w111 -> [w316]
    tunnel: w109 -> [w315] mode=indexing
    tunnel: w108 -> [w314] mode=indexing
    tunnel: w107 -> [w313] mode=indexing
    tunnel: w106 -> [w312] mode=indexing
    tunnel: w105 -> [w311] mode=indexing
    tunnel: w104 -> [w310] mode=indexing
    tunnel: [w309] -> w93 mode=indexing
    tunnel: [w308] -> w92 mode=indexing
    n102 = for {
      tunnel: w317 -> [w326] mode=indexing
      tunnel: w316 -> [w336]
      tunnel: w315 -> [w325]
      tunnel: w314 -> [w324]
      tunnel: w313 -> [w323]
      tunnel: w312 -> [w322]
      tunnel: w311 -> [w321]
      tunnel: w310 -> [w320]
      tunnel: [w319] -> w309 mode=indexing
      tunnel: [w318] -> w308 mode=indexing
      n103 = Index Array(array=w326, index=0) -> (element=w335:dbl)
      n104 = Index Array(array=w326, index=3) -> (element=w327:dbl)
      n105 = Unbundle By Name(w336) -> ("A"=w334:dbl, "B"=w333:dbl, "n"=w332:dbl, "A"=w331:dbl, "B"=w330:dbl, "n"=w329:dbl)
      n106 = formula code="float64 tana, tana2, Urefcosa ;\n\na *= pi / 180.0 ;\ntana = tan(a) ;\nUrefcosa = Uref * cos(a) ;\n\ntana2 = tana * tana ;\nUrefcosa *= Urefcosa ;\n\nE1H = sqrt(A1 + B1 * (((1.0 - (a1H * tana2) - (b1H * tana) - c1H) * Urefcosa)**(0.5 * n1))) ;\nE2H = sqrt(A2 + B2 * (((1.0 - (a2H * tana2) - (b2H * tana) - c2H) * Urefcosa)**(0.5 * n2))) ;"("A1"=w334, "B1"=w333, "n1"=w332, "A2"=w331, "B2"=w330, "n2"=w329, "a"=w335, "Uref"=w327, "a1H"=w325, "a2H"=w324, "b1H"=w323, "b2H"=w322, "c1H"=w321, "c2H"=w320) -> ("E1H"=w319:dbl, "E2H"=w318:dbl)
    }
  }
  n107 = Array Size(array=w110) -> (size(s)=w155:i32[])
  n108 = Index Array(array=w155, index=0) -> (element=→"Angle sets":i32)
  n109 = for {
    shift-right: [w353] -> w117
    shift-left: cluster{dbl[], dbl[]}[] [] -> [w350]
    tunnel: w110 -> [w354] mode=indexing
    tunnel: [w360] -> w116 mode=indexing
    tunnel: [w358] -> w1 mode=indexing
    shift-right: [w346] -> w59
    shift-left: w45 -> [w349]
    shift-right: [w348] -> w73
    shift-left: w45 -> [w347]
    shift-right: [w338] -> w71
    shift-left: w45 -> [w343]
    tunnel: w92 -> [w342] mode=indexing
    tunnel: w93 -> [w341] mode=indexing
    shift-right: [w340] -> w72
    shift-left: w45 -> [w339]
    n110 = Index Array(array=w354, index (col)=0 ("index")) -> (element=w360:dbl[])  [unwired: 1 in]
    n111 = Index Array(array=w354, index (col)=3 ("index")) -> (element=w359:dbl[])  [unwired: 1 in]
    n112 = Index Array(array=w354, index (col)=1 ("index")) -> (element=w345:dbl[])  [unwired: 1 in]
    n113 = Index Array(array=w354, index (col)=2 ("index")) -> (element=w344:dbl[])  [unwired: 1 in]
    n114 = call <vilib>:"Mean.vi"("X"=w359) -> ("mean"=w358:dbl)  [unwired: 1 out]
    n115 = Bundle(w345, w344) -> (w351:cluster{dbl[], dbl[]})  [unwired: 1 out]
    n116 = Build Array (concatenate)(w350, w351) -> (w353:cluster{dbl[], dbl[]}[])
    n117 = Build Array (concatenate)(w345, w347) -> (w348:dbl[])
    n118 = Build Array (concatenate)(w344, w349) -> (w346:dbl[])
    n119 = Build Array (concatenate)(w341, w339) -> (w340:dbl[])
    n120 = Build Array (concatenate)(w342, w343) -> (w338:dbl[])
  }
  "Uref associated with each angle set (m/s)" <- w1
  "E1', E2' map coloured by angle set" <- w117
  n121 = Less?(x=w22, y=0) -> (x < y?=w29:bool)
  n122 = Bundle(w73, w59) -> (w113:cluster{dbl[], dbl[]})  [unwired: 1 out]
  n123 = Bundle(w72, w71) -> (w91:cluster{dbl[], dbl[]})  [unwired: 1 out]
  n124 = Build Array(w73, w59, w72, w71) -> (w70:dbl[][])
  n125 = Transpose 2D Array(2D array=w116) -> (transposed array=→"Probe angles traversed in each angle set\n1st index: angle (deg)\n2nd index: angle set":dbl[][])
  n126 = Transpose 2D Array(2D array=w70) -> (transposed array=w68:dbl[][])
  n127 = Build Array(w113, w91) -> (→"E1', E2' map synthesized from effective angle methods LS fits":cluster{dbl[], dbl[]}[])
  n128 = Array To Spreadsheet String(array=w68, 3:"%.16f" ("format string")) -> (spreadsheet string=w61:string)  [unwired: 1 out]
  n129 = case shown="False" w29 {
    tunnel: w89 -> [w374 w381]
    tunnel: w88 -> [w373 w378]
    tunnel: [w363 w379] -> w90
    tunnel: w22 -> [w372 _]
    tunnel: w49 -> [w371 w375]
    tunnel: w48 -> [w370 w376]
    tunnel: w47 -> [w369 w377]
    frame False {
      n130 = Index Array(array=w374, index=w372) -> (element=w361:cluster{dbl[], "P(A)":dbl[]})
      n131 = Index Array(array=w373, index=w372) -> (element=w362:cluster{dbl[], "P(A)":dbl[]})
      n132 = Index Array(array=w371, index (row)=w372) -> (element=w366:dbl[])  [unwired: 1 in]
      n133 = Index Array(array=w370, index (row)=w372) -> (element=w365:dbl[])  [unwired: 1 in]
      n134 = Index Array(array=w369, index (row)=w372) -> (element=w364:dbl[])  [unwired: 1 in]
      n135 = Bundle(w366, w365) -> (w367:cluster{dbl[], dbl[]})  [unwired: 1 out]
      n136 = Bundle(w366, w364) -> (w368:cluster{dbl[], dbl[]})  [unwired: 1 out]
      n137 = Build Array(w367, w368, w361, w362) -> (w363:cluster{dbl[], "P(A)":dbl[]}[])
    }
    frame True {
      n138 = for {
        tunnel: w381 -> [w387] mode=indexing
        tunnel: w378 -> [w388] mode=indexing
        shift-right: [w390] -> w379
        shift-left: cluster{dbl[], dbl[]}[] [] -> [w389]
        tunnel: w377 -> [w384] mode=indexing
        tunnel: w376 -> [w385] mode=indexing
        tunnel: w375 -> [w386] mode=indexing
        n139 = Bundle(w386, w385) -> (w383:cluster{dbl[], dbl[]})  [unwired: 1 out]
        n140 = Bundle(w386, w384) -> (w382:cluster{dbl[], dbl[]})  [unwired: 1 out]
        n141 = Build Array (concatenate)(w389, w383, w382, w387, w388) -> (w390:cluster{dbl[], "P(A)":dbl[]}[])
      }
    }
  }
  "Effective angle X plot_" <- w90
  n142 = for {
    tunnel: w49 -> [w396] mode=indexing
    tunnel: w48 -> [w395] mode=indexing
    tunnel: w47 -> [w394] mode=indexing
    shift-right: [w399] -> w53
    shift-left: "" -> [w398]
    shift-right: [w392] -> w54
    shift-left: dbl[][] [] -> [w391]
    i -> [w405]
    w400 = "\t"
    n143 = Number To Decimal String(number=w405) -> (decimal integer string=w401:string)  [unwired: 1 out]
    n144 = Build Array (concatenate)(w391, w396, w395, w394, dbl[] [] ("element")) -> (w392:dbl[][])
    n145 = Concatenate Strings("x_" ("format string"), w401, w400, "y1_" ("format string"), w401, w400, "y2_" ("format string"), w401, w400, w400) -> (w397:string)
    n146 = Concatenate Strings(w398, w397) -> (w399:string)
  }
  n147 = Array Size(array=w2) -> (size(s)=w5:i32)
  n148 = Decrement(x=w5) -> (x-1=w6:i32)
  n149 = while {
    shift-right: [w423] -> w12
    shift-left: w20 -> [w426]
    shift-right: [w424] -> w13
    shift-left: w19 -> [w425]
    shift-right: [w421] -> w4
    shift-left: w18 -> [w422]
    shift-right: [w413] -> w11
    shift-left: w17 -> [w420]
    shift-right: [w414] -> w10
    shift-left: w16 -> [w419]
    shift-right: [w415] -> w9
    shift-left: w15 -> [w418]
    shift-right: [w416] -> w8
    shift-left: w14 -> [w417]
    shift-right: [w411] -> w7
    shift-left: w1 -> [w412]
    shift-right: [w406] -> _
    shift-left: w6 -> [w407]
    tunnel: w2 -> [w410]
    stop <- w409 stop-if-true
    n150 = Index Array(array=w410, index=w407) -> (element=w408:bool)
    n151 = case shown="True" w408 {
      tunnel: [w434 w450] -> w423
      tunnel: w426 -> [w434 w451]
      tunnel: w425 -> [w433 w449]
      tunnel: [w433 w448] -> w424
      tunnel: w422 -> [w432 w447]
      tunnel: [w432 w446] -> w421
      tunnel: w420 -> [w428 w441]
      tunnel: w419 -> [w429 w442]
      tunnel: w418 -> [w430 w443]
      tunnel: w417 -> [w431 w445]
      tunnel: [w431 w444] -> w416
      tunnel: [w430 w438] -> w415
      tunnel: [w429 w439] -> w414
      tunnel: [w428 w440] -> w413
      tunnel: w412 -> [w427 w437]
      tunnel: [w427 w436] -> w411
      tunnel: w407 -> [_ w435]
      frame False {
      }
      frame True {
        n152 = Delete From Array(array=w449, index=w435) -> (array with subset deleted=w448:dbl[])  [unwired: 1 in, 1 out]
        n153 = Delete From Array(array=w441, index=w435) -> (array with subset deleted=w440:dbl[])  [unwired: 1 in, 1 out]
        n154 = Delete From Array(array=w442, index=w435) -> (array with subset deleted=w439:dbl[])  [unwired: 1 in, 1 out]
        n155 = Delete From Array(array=w443, index=w435) -> (array with subset deleted=w438:dbl[])  [unwired: 1 in, 1 out]
        n156 = Delete From Array(array=w445, index=w435) -> (array with subset deleted=w444:dbl[])  [unwired: 1 in, 1 out]
        n157 = Delete From Array(array=w437, index=w435) -> (array with subset deleted=w436:dbl[])  [unwired: 1 in, 1 out]
        n158 = Delete From Array(array=w451, index=w435) -> (array with subset deleted=w450:dbl[])  [unwired: 1 in, 1 out]
        n159 = Delete From Array(array=w447, index=w435) -> (array with subset deleted=w446:dbl[])  [unwired: 1 in, 1 out]
      }
    }
    n160 = Decrement(x=w407) -> (x-1=w406:i32)
    n161 = Less Than 0?(x=w406) -> (x < 0?=w409:bool)
  }
  n162 = Concatenate Strings("E1' actual data (Volts)", w67, "E2' actual data (Volts)", w67, "E1' higher order eff. angle method (Volts)", w67, "E2' higher order eff. angle method (Volts)", "\r", w61) -> (→"E1, E2 maps for each method":string)
  n163 = Multiply(x=w22, y=2) -> (x*y=w21:i32)
  n164 = Transpose 2D Array(2D array=w54) -> (transposed array=w56:dbl[][])
  n165 = call <vilib>:"Trim Whitespace.vi"("string"=w53) -> ("trimmed string"=w52:string)  [unwired: 1 in]
  n166 = Bundle(w7, w12) -> (w101:cluster{dbl[], dbl[]})  [unwired: 1 out]
  n167 = Bundle(w7, w4) -> (w100:cluster{dbl[], dbl[]})  [unwired: 1 out]
  n168 = Bundle(w7, w11) -> (w98:cluster{dbl[], dbl[]})  [unwired: 1 out]
  n169 = Bundle(w7, w10) -> (w99:cluster{dbl[], dbl[]})  [unwired: 1 out]
  n170 = Bundle(w7, w13) -> (→"Probe zero alignment error_":cluster{dbl[], dbl[]})  [unwired: 1 out]
  n171 = Bundle(w7, w9) -> (w96:cluster{dbl[], dbl[]})  [unwired: 1 out]
  n172 = Bundle(w7, w8) -> (w95:cluster{dbl[], dbl[]})  [unwired: 1 out]
  n173 = case shown="False" w29 {
    tunnel: w30 -> [w455 w456]
    tunnel: w21 -> [w454 _]
    tunnel: [w452 w456] -> w28
    frame False {
      n174 = Array Subset(array=w455, index=w454, length=2) -> (w452:cluster{dbl[], dbl[]}[])
    }
    frame True {
    }
  }
  "Quartic tan(2e) function" <- w28
  n175 = Array To Spreadsheet String(array=w56, 3:"%.16f" ("format string")) -> (spreadsheet string=w50:string)  [unwired: 1 out]
  n176 = Build Array(w101, w100) -> (→"Wire angle error with speed_":cluster{dbl[], dbl[]}[])
  n177 = Build Array(w98, w99) -> (→"Effective angle variation with speed_":cluster{dbl[], dbl[]}[])
  n178 = Build Array(w96, w95) -> (→"Variation of tangential cooling coefficient k with speed":cluster{dbl[], dbl[]}[])
  n179 = Build Array(w7, w12, w4, w13, w11, w10, w9, w8) -> (w87:dbl[][])
  n180 = Concatenate Strings(w52, "\r", w50) -> (→"Higher order effective angle method X plot data (each angle set separated by a column of zeros)":string)
  n181 = Transpose 2D Array(2D array=w87) -> (transposed array=w3:dbl[][])
  n182 = Array To Spreadsheet String(array=w3, 3:"%.16f" ("format string")) -> (spreadsheet string=w75:string)  [unwired: 1 out]
  n183 = Concatenate Strings("Uref (m/s)", w78, "eps1 (deg)", w78, "eps2 (deg)", w78, "Probe zero err. (deg)", w78, "theta 1 (deg)", w78, "theta 2 (deg)", w78, "k1", w78, "k2", "\r", w75) -> (→"Quantities that vary with Uref (epsilon, theta, k) (higher order method)":string)
  n184 = Transpose 2D Array(2D array=w35) -> (transposed array=→"Roots for e1 (2nd index angle set- 1)":cdb[][])
  n185 = Transpose 2D Array(2D array=w32) -> (transposed array=→"Roots for e2 (2nd index angle set -1)":cdb[][])
